vi "NIMS_NS_fir_linf.vi"(5 "Function name":string, 6 "Line number":i32, 7 "Number of outputs requested":i32, 8 "error in (no error)":errorcluster, 11 "[A]":variant[](array[variant])) -> (0 "error out":errorcluster, 3 "[funct(A)]":variant[](array[variant]))   [LabVIEW 2017]
uses:
  <vilib>/imath/engines/lvmath/Functions/Error Handling/error.ctl
  <instcachedir>/0/NIMS_RunTimeType_From StrictType (excl LVString)_1019F277F0A747EDBCA0F6C52CA54500.lvgen/NIMS_RunTimeType_From StrictType (excl LVString)_1019F277F0A747EDBCA0F6C52CA54500_000.vi
  <instcachedir>/0/NIMS_Get Scalar_w Error_1987D997E87247DDAC16EA23A5E9E4FC.lvgen/NIMS_Get Scalar_w Error_1987D997E87247DDAC16EA23A5E9E4FC_000.vi
  <instcachedir>/0/NIMS_Get Any Vector_w Error - Matrix_9FDB8FBE264C42EDBC8FF9BA66C3EF33.lvgen/NIMS_Get Any Vector_w Error - Matrix_9FDB8FBE264C42EDBC8FF9BA66C3EF33_001.vi
  <instcachedir>/0/NIMS_Complex To Real_BE01396FDE034E8E94CEBBA1E368668D.lvgen/NIMS_Complex To Real_BE01396FDE034E8E94CEBBA1E368668D_000.vi
  <instcachedir>/0/NIMS_Get Row Vector_w Error - Matrix_7ECCFA0649AF47C08F6F0C496599EB01.lvgen/NIMS_Get Row Vector_w Error - Matrix_7ECCFA0649AF47C08F6F0C496599EB01_000.vi
  <instcachedir>/0/NIMS_RunTimeType_To Numeric_1CBDAFC4EFAD4045A1DE52278D16738D.lvgen/NIMS_RunTimeType_To Numeric_1CBDAFC4EFAD4045A1DE52278D16738D_000.vi
  <vilib>/addons/Digital Filter Design/NI_DigFilter_MathScript.lvlib
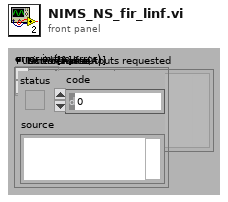
[diagram p1: front panel]
types:
  T1 = typedef "error.ctl" = enum16{"No Error", "Problem", "Input type must not be void", "Incorrect number of parameters", "Function not defined for non-numeric types", "An output variable of the user-defined function is undefined", "Function only defined for character arrays", "Function not defined for boolean, character, or single precision", "Function not defined for complex types", "Not a valid operation", "Inputs must be scalar", "Input matrices are not the same size", "Function only available on RT", "Input matrices must be nonnegative integers of the same type", "Arguments must be non-negative integers less than bitmax", "Number to complement must be less than 2^N", "Bit to get is outside range", "Bit to set is outside range", "Input must be real type ", "At least one parameter must be scalar", "Unable to display plug-in data on RT", "Function not defined for higher dimensional matrices", "Invalid attributes", "Wrong Type of Input Arguments", "Wrong Argument Option", "Invalid file identifier", "Indices must be real positive integers", "The variable is not a matrix data type.", "Number of elements must be the same for indices and values", "You cannot replace elements of a matrix with non-matrix data types.", "Cannot resize a 2D matrix with a linear index", "Unknown variable or symbol", "Indices out of range", "Empty matrix deletion can not be used with two indices", "Number of rows and columns must be the same for indices and values.", "Complex cannot be converted to Boolean", "Char cannot be converted to Boolean", "int64 cannot be converted to Boolean", "uint64 cannot be converted to Boolean", "You cannot convert a Boolean to a character.", "Incompatible input size in 3D surface function", "All rows must have the same number of columns", "Incompatible types", "Invalid matrix dimensions", "Dimension must be 1 or 2", "Base must be an integer between 2 and 36", "Invalid input", "Square matrix required", "Function 'timerstart' must be called before 'timerstop'", "Arguments must be positive real", "Step must not be zero", "Wrong number of input arguments", "Wrong number of output arguments", "Too many index arguments", "Input scalar must be >= 0", "Input scalar must be positive", "Input scalar must not be 0", "Input scalar must be in range [0,1]", "Can't use conditionally defined variable that's undefined", "Input must be a vector", "RT Exec Trace Toolkit not licensed", "Empty vector error", "All elements must be in domain [-1,1]", "All real elements of input vector must be >= 0", "All elements of input vector must be positive", "Values of input vectors are not compatible", "DAQmx not installed", "Input vector must be an increasing vector", "Dereferenced field does not exist within the struct", "A vector or matrix of structures must be indexed before it can be dereferenced", "Lenths of two input vectors are not compatible", "Invalid fieldname", "Empty matrix error", "Cannot use '.' on a type other than Struct", "Unused074", "Data type of the struct's field name is invalid", "Using . to dereference data that is not a struct", "Input struct contains invalid type ", "Size of input matrix is incompatible with input size", "Invalid format specifier", "Could not find field within struct", "Bad permutation array", "Mismatched fieldnames", "ode: User Function could not be opened", "ode: User Function signature does not meet ode requirements", "Unused085", "RunTime: MathScript could not be compiled", "Unknown function", "Only scalars and strings supported", "ode: User Function signature has incorrect number of inputs", "ode:User Function signature has incorrect number of outputs", "Range is too large", "End used without variable", "Function not available (RTE)", "Custom user error", "Arguments must be integers less than bitmax", "Shared library not found", "Header file not found", "Shared library already loaded", "Shared library not loaded", "Shared library function not found", "Shared library string return problem", "Problem calling shared library function", "Problem loading shared library from OS", "Problem parsing shared library header file", "Shared library incompatible types", "Shared library unsupported return type", "Shared library function not exported", "Shared library unsupported input type", "Problem unloading shared library from OS", "Function only available from UI", "Function specified in argument is missing", "An internal error has occurred", "Invalid object", "Invalid property", "Read-only property", "A break command has occurred", "A continue command has occurred", "A return command has occurred", "ode: times parameter invalid", "Function specified in argument has incorrect signature", "Function not found in file", "Reserved keyword cannot be defined as variable", "Reserved keyword cannot be defined as a function or script", "Arguments must be string literals", "Function not supported on this platform", "All columns must have the same number of rows", "Function ignored in RTE warning", "Cannot use : as a parameter that is not a variable", "Output can't be coerced to requested type", "Function not supported on current target", "Variable dependent on an unwired function input", "Unused132", "Unused133", "Unused134", "Unused135", "Unused136", "Unused137", "Unused138", "Unused139", "Global/Persistent must only take constants as arguments.", "Varargin must be last input in the function definition.", "Varargout must be last output in the function definition.", "Invalid output type. Cannot output a cell array of any type other than string.", "Invalid output type. Type is a dynamic struct.", "Invalid output type. Type is a struct that has a field whose type is not known until run-time", "Invalid output type. Type is a struct that has a field which is a plot object.", "MathScript parser DLL missing", "MathScript requires LabVIEW Full", "MathScript license is invalid or missing", "Varargout not supported except in assignments."}
  T2 = typedef "NIMS_CH_character datatype.ctl" = cluster{"Numeric":u8}
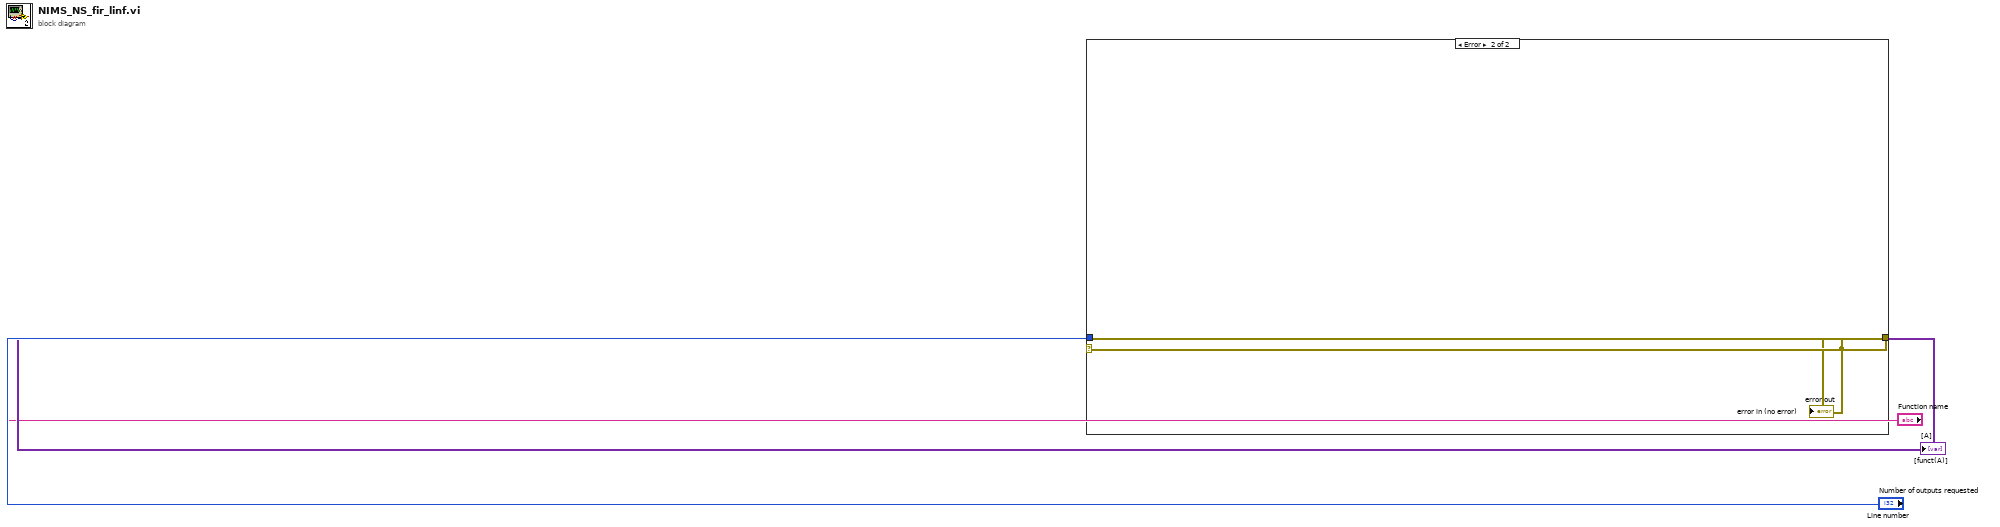
[diagram p0: block diagram]
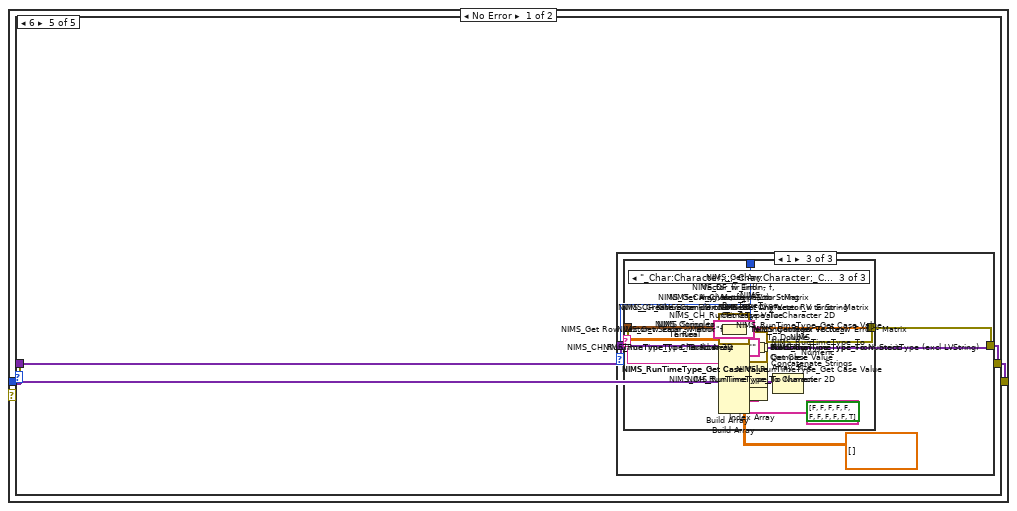
[diagram p2: hidden frame]
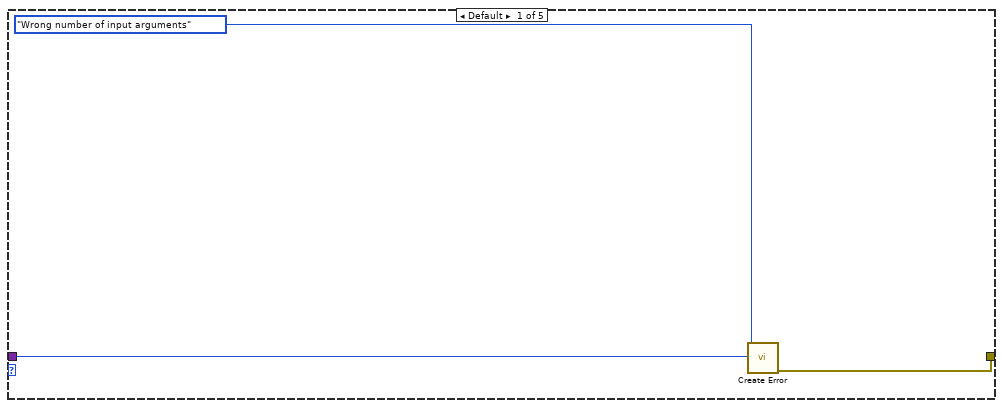
[diagram p3: hidden frame]
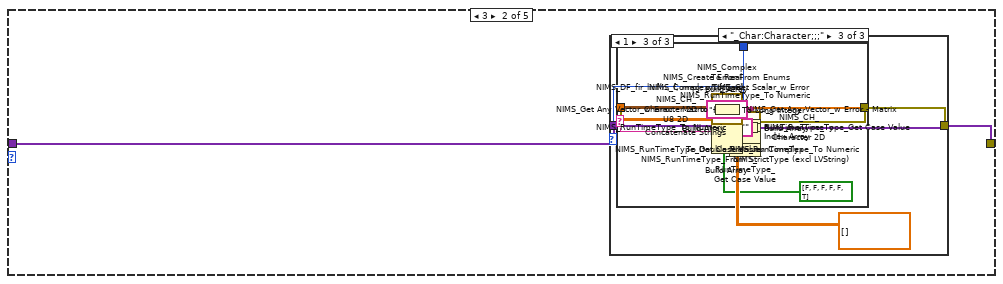
[diagram p4: hidden frame]
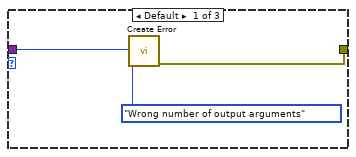
[diagram p5: hidden frame]
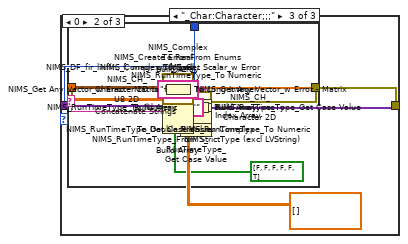
[diagram p6: hidden frame]
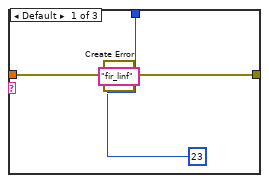
[diagram p7: hidden frame]
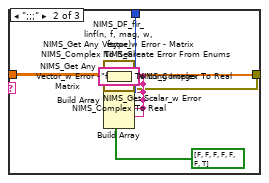
[diagram p8: hidden frame]
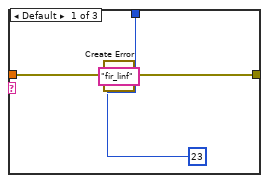
[diagram p9: hidden frame]
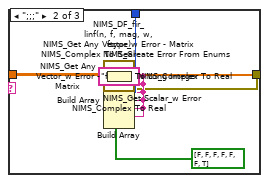
[diagram p10: hidden frame]
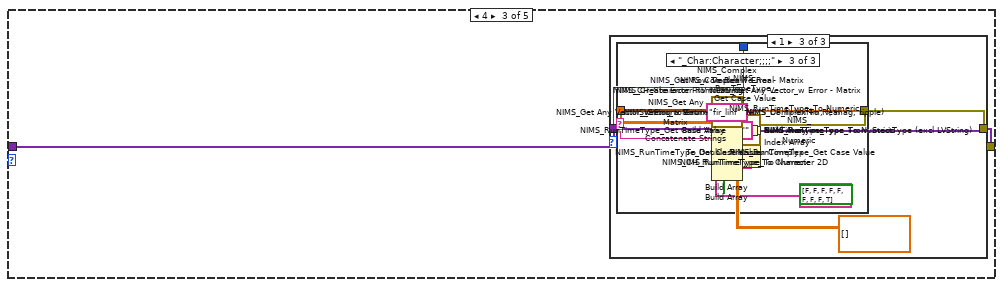
[diagram p11: hidden frame]
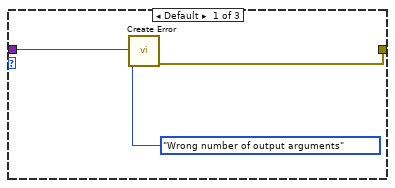
[diagram p12: hidden frame]
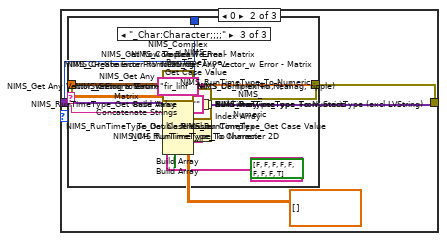
[diagram p13: hidden frame]
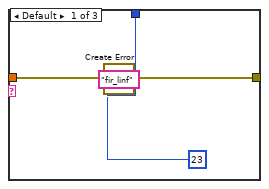
[diagram p14: hidden frame]
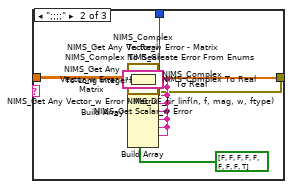
[diagram p15: hidden frame]
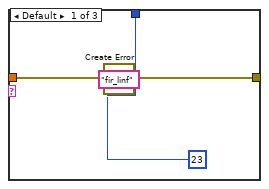
[diagram p16: hidden frame]
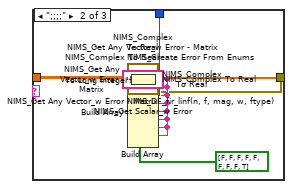
[diagram p17: hidden frame]
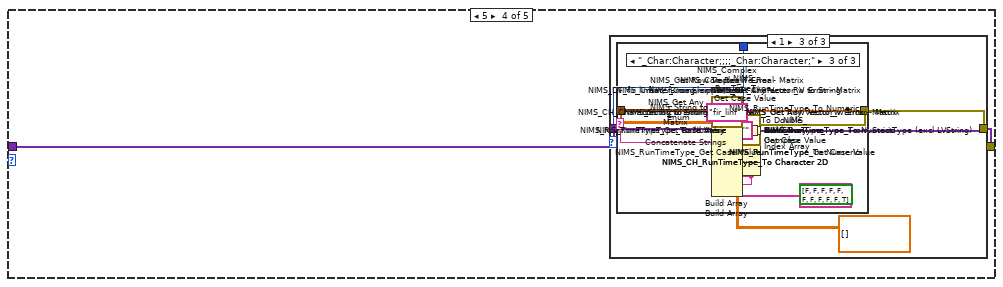
[diagram p18: hidden frame]
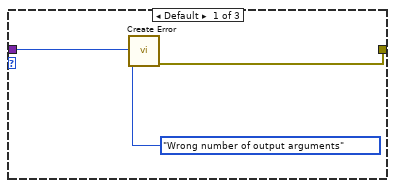
[diagram p19: hidden frame]
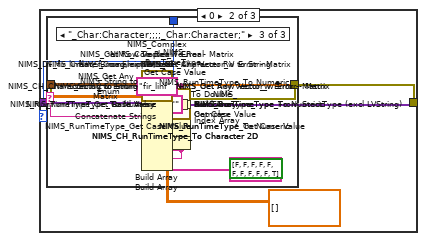
[diagram p20: hidden frame]
diagram:
  n1 = case shown="Error" "error in (no error)" {
    selector: "error in (no error)" -> [_ w885]
    tunnel: [w15 _] -> w4
    tunnel: [w14 w885] -> w3
    tunnel: "error in (no error)" -> [w13 _]
    tunnel: "Number of outputs requested" -> [w12 _]
    tunnel: "[A]" -> [w11 _]
    tunnel: "Function name" -> [w10 _]
    tunnel: "Line number" -> [w9 _]
    frame No Error {
      n2 = Array Size(array=w11) -> (size(s)=w8:i32)
      n3 = case shown="6" w8 {
        tunnel: [_ w27 w199 w403 w635] -> w15
        tunnel: w10 -> [w19 w24 w196 w400 w632]
        tunnel: w9 -> [w20 w25 w197 w401 w633]
        tunnel: w13 -> [w17 w23 w195 w399 w631]
        tunnel: [w16 w22 w194 w398 w630] -> w14
        tunnel: w12 -> [_ w21 w193 w397 w629]
        tunnel: w11 -> [_ w26 w198 w402 w634]
        frame Default {
          n4 = call <vilib>:"Create Error.vi"("Function name"=w19, "error in (no error)"=w17, "Error Enum"=error."Wrong number of input arguments", "Line number"=w20) -> ("error out"=w16:errorcluster)  [unwired: 6 in, 1 out]
        }
        frame 3 {
          n5 = case shown="1" w21 {
            tunnel: [_ w33 w113] -> w27
            tunnel: w24 -> [w31 _ _]
            tunnel: w25 -> [w32 w55 w135]
            tunnel: w23 -> [w29 w53 w133]
            tunnel: [w28 w39 w119] -> w22
            tunnel: w26 -> [_ w56 w136]
            frame Default {
              n6 = call <vilib>:"Create Error.vi"("Function name"=w31, "error in (no error)"=w29, "Error Enum"=error."Wrong number of output arguments", "Line number"=w32) -> ("error out"=w28:errorcluster)  [unwired: 6 in, 1 out]
            }
            frame 0 {
              n7 = Index Array(array=w56) -> (element #1=w52:variant, element #2=w47:variant, element #3=w43:variant)  [unwired: 3 in]
              n8 = call <vilib>:"NIMS_RunTimeType_Get Case Value.vi"("Data In"=w43) -> ("Case Value"=w40:string)  [unwired: 9 in, 1 out]
              n9 = call-generic <vilib>:"NIMS_RunTimeType_To Numeric.vi"("DataType"=cdb[][] [], "Variant"=w43) -> ("data"=w41:cdb[][])  [unwired: 1 in]
              n10 = call <vilib>:"NIMS_RunTimeType_Get Case Value.vi"("Data In"=w47) -> ("Case Value"=w44:string)  [unwired: 9 in, 1 out]
              n11 = call-generic <vilib>:"NIMS_RunTimeType_To Numeric.vi"("DataType"=cdb[][] [], "Variant"=w47) -> ("data"=w45:cdb[][])  [unwired: 1 in]
              n12 = call <vilib>:"NIMS_RunTimeType_Get Case Value.vi"("Data In"=w52) -> ("Case Value"=w48:string)  [unwired: 9 in, 1 out]
              n13 = call <vilib>:"NIMS_CH_RunTimeType_To Character 2D.vi"("Variant"=w52) -> ("data"=w49:T2[][])  [unwired: 1 in]
              n14 = call-generic <vilib>:"NIMS_RunTimeType_To Numeric.vi"("DataType"=cdb[][] [], "Variant"=w52) -> ("data"=w50:cdb[][])  [unwired: 1 in]
              n15 = Concatenate Strings(w48, w44, w40) -> (w54:string)
              n16 = case shown="\"_Char:Character;;;\"" w54 {
                tunnel: w53 -> [w58 w67 w93]
                tunnel: [_ w62 w88] -> w38
                tunnel: [w57 w63 w89] -> w39
                tunnel: w50 -> [_ w86 _]
                tunnel: w49 -> [_ _ w111]
                tunnel: w45 -> [_ w82 w107]
                tunnel: w41 -> [_ w79 w104]
                tunnel: w55 -> [w61 w70 w96]
                frame Default {
                  n17 = call <vilib>:"Create Error.vi"("Function name"="fir_linf", "error in (no error)"=w58, "Error Enum"=23, "Line number"=w61) -> ("error out"=w57:errorcluster)  [unwired: 6 in, 1 out]
                }
                frame ";;;" {
                  w65 = "fir_linf"
                  n18 = call-generic <vilib>:"NIMS_Complex To Real.vi"("A"=w79) -> ("Error Enum"=w73:T1, "Real(A)"=w78:dbl[][])  [unwired: 8 in, 1 out]
                  n19 = call-generic <vilib>:"NIMS_Get Any Vector_w Error - Matrix.vi"("A"=w78) -> ("Error Enum"=w72:T1, "Vector"=w80:dbl[])  [unwired: 8 in, 1 out]
                  n20 = call-generic <vilib>:"NIMS_Complex To Real.vi"("A"=w82) -> ("Error Enum"=w75:T1, "Real(A)"=w81:dbl[][])  [unwired: 8 in, 1 out]
                  n21 = call-generic <vilib>:"NIMS_Get Any Vector_w Error - Matrix.vi"("A"=w81) -> ("Error Enum"=w74:T1, "Vector"=w83:dbl[])  [unwired: 8 in, 1 out]
                  n22 = call-generic <vilib>:"NIMS_Complex To Real.vi"("A"=w86) -> ("Error Enum"=w77:T1, "Real(A)"=w85:dbl[][])  [unwired: 8 in, 1 out]
                  n23 = To Long Integer(number=w85) -> (32bit integer=w84:i32[][])
                  n24 = call-generic <vilib>:"NIMS_Get Scalar_w Error.vi"("A"=w84) -> ("Error Enum"=w76:T1, "Scalar"=w87:i32)  [unwired: 8 in, 1 out]
                  n25 = call <vilib>:"NIMS_DF_fir_linf(n, f, mag, w, ftype).vi"("mag"=w80, "f"=w83, "n"=w87) -> ("error"=w71:i32, "b"=w62:dbl[])  [unwired: 7 in]
                  n26 = Build Array(w65, w65, w65, w65, w65, w65, "fir_linf") -> (w68:string[])
                  n27 = Build Array(w77, w76, w75, w74, w73, w72, w71) -> (w69:i32[])
                  n28 = call <vilib>:"NIMS_Create Error From Enums.vi"("Error Code"=bool[] [FALSE, FALSE, FALSE, FALSE, FALSE, FALSE, TRUE], "error in (no error)"=w67, "Line no"=w70, "Error Enums"=w69, "Function names"=w68) -> ("error out"=w63:errorcluster)  [unwired: 6 in]
                }
                frame "_Char:Character;;;" {
                  w91 = "fir_linf"
                  n29 = call-generic <vilib>:"NIMS_Complex To Real.vi"("A"=w104) -> ("Error Enum"=w99:T1, "Real(A)"=w103:dbl[][])  [unwired: 8 in, 1 out]
                  n30 = call-generic <vilib>:"NIMS_Get Any Vector_w Error - Matrix.vi"("A"=w103) -> ("Error Enum"=w98:T1, "Vector"=w105:dbl[])  [unwired: 8 in, 1 out]
                  n31 = call-generic <vilib>:"NIMS_Complex To Real.vi"("A"=w107) -> ("Error Enum"=w101:T1, "Real(A)"=w106:dbl[][])  [unwired: 8 in, 1 out]
                  n32 = call-generic <vilib>:"NIMS_Get Any Vector_w Error - Matrix.vi"("A"=w106) -> ("Error Enum"=w100:T1, "Vector"=w108:dbl[])  [unwired: 8 in, 1 out]
                  n33 = call <vilib>:"NIMS_CH_Character 2D to U8 2D.vi"("Character 2D array"=w111) -> ("U8 2D array"=w110:u8[][])  [unwired: 10 in]
                  n34 = To Long Integer(number=w110) -> (32bit integer=w109:i32[][])
                  n35 = call-generic <vilib>:"NIMS_Get Scalar_w Error.vi"("A"=w109) -> ("Error Enum"=w102:T1, "Scalar"=w112:i32)  [unwired: 8 in, 1 out]
                  n36 = call <vilib>:"NIMS_DF_fir_linf(n, f, mag, w, ftype).vi"("mag"=w105, "f"=w108, "n"=w112) -> ("error"=w97:i32, "b"=w88:dbl[])  [unwired: 7 in]
                  n37 = Build Array(w91, w91, w91, w91, w91, "fir_linf") -> (w94:string[])
                  n38 = Build Array(w102, w101, w100, w99, w98, w97) -> (w95:i32[])
                  n39 = call <vilib>:"NIMS_Create Error From Enums.vi"("Error Code"=bool[] [FALSE, FALSE, FALSE, FALSE, FALSE, TRUE], "error in (no error)"=w93, "Line no"=w96, "Error Enums"=w95, "Function names"=w94) -> ("error out"=w89:errorcluster)  [unwired: 6 in]
                }
              }
              n40 = Build Array(w38) -> (w37:dbl[][])
              n41 = To Double Precision Complex(1:w37) -> (0:w36:cdb[][])
              n42 = call-generic <vilib>:"NIMS_RunTimeType_From StrictType (excl LVString).vi"("Plug-In Name"="", "Data In"=w36) -> ("Data Out"=w34:variant)  [unwired: 2 in]
              n43 = Build Array(w34) -> (w33:variant[])
            }
            frame 1 {
              n44 = Index Array(array=w136) -> (element #1=w132:variant, element #2=w127:variant, element #3=w123:variant)  [unwired: 3 in]
              n45 = call <vilib>:"NIMS_RunTimeType_Get Case Value.vi"("Data In"=w123) -> ("Case Value"=w120:string)  [unwired: 9 in, 1 out]
              n46 = call-generic <vilib>:"NIMS_RunTimeType_To Numeric.vi"("DataType"=cdb[][] [], "Variant"=w123) -> ("data"=w121:cdb[][])  [unwired: 1 in]
              n47 = call <vilib>:"NIMS_RunTimeType_Get Case Value.vi"("Data In"=w127) -> ("Case Value"=w124:string)  [unwired: 9 in, 1 out]
              n48 = call-generic <vilib>:"NIMS_RunTimeType_To Numeric.vi"("DataType"=cdb[][] [], "Variant"=w127) -> ("data"=w125:cdb[][])  [unwired: 1 in]
              n49 = call <vilib>:"NIMS_RunTimeType_Get Case Value.vi"("Data In"=w132) -> ("Case Value"=w128:string)  [unwired: 9 in, 1 out]
              n50 = call <vilib>:"NIMS_CH_RunTimeType_To Character 2D.vi"("Variant"=w132) -> ("data"=w129:T2[][])  [unwired: 1 in]
              n51 = call-generic <vilib>:"NIMS_RunTimeType_To Numeric.vi"("DataType"=cdb[][] [], "Variant"=w132) -> ("data"=w130:cdb[][])  [unwired: 1 in]
              n52 = Concatenate Strings(w128, w124, w120) -> (w134:string)
              n53 = case shown="\"_Char:Character;;;\"" w134 {
                tunnel: w133 -> [w138 w147 w173]
                tunnel: [_ w142 w168] -> w118
                tunnel: [w137 w143 w169] -> w119
                tunnel: w130 -> [_ w166 _]
                tunnel: w129 -> [_ _ w191]
                tunnel: w125 -> [_ w162 w187]
                tunnel: w121 -> [_ w159 w184]
                tunnel: w135 -> [w141 w150 w176]
                frame Default {
                  n54 = call <vilib>:"Create Error.vi"("Function name"="fir_linf", "error in (no error)"=w138, "Error Enum"=23, "Line number"=w141) -> ("error out"=w137:errorcluster)  [unwired: 6 in, 1 out]
                }
                frame ";;;" {
                  w145 = "fir_linf"
                  n55 = call-generic <vilib>:"NIMS_Complex To Real.vi"("A"=w159) -> ("Error Enum"=w153:T1, "Real(A)"=w158:dbl[][])  [unwired: 8 in, 1 out]
                  n56 = call-generic <vilib>:"NIMS_Get Any Vector_w Error - Matrix.vi"("A"=w158) -> ("Error Enum"=w152:T1, "Vector"=w160:dbl[])  [unwired: 8 in, 1 out]
                  n57 = call-generic <vilib>:"NIMS_Complex To Real.vi"("A"=w162) -> ("Error Enum"=w155:T1, "Real(A)"=w161:dbl[][])  [unwired: 8 in, 1 out]
                  n58 = call-generic <vilib>:"NIMS_Get Any Vector_w Error - Matrix.vi"("A"=w161) -> ("Error Enum"=w154:T1, "Vector"=w163:dbl[])  [unwired: 8 in, 1 out]
                  n59 = call-generic <vilib>:"NIMS_Complex To Real.vi"("A"=w166) -> ("Error Enum"=w157:T1, "Real(A)"=w165:dbl[][])  [unwired: 8 in, 1 out]
                  n60 = To Long Integer(number=w165) -> (32bit integer=w164:i32[][])
                  n61 = call-generic <vilib>:"NIMS_Get Scalar_w Error.vi"("A"=w164) -> ("Error Enum"=w156:T1, "Scalar"=w167:i32)  [unwired: 8 in, 1 out]
                  n62 = call <vilib>:"NIMS_DF_fir_linf(n, f, mag, w, ftype).vi"("mag"=w160, "f"=w163, "n"=w167) -> ("error"=w151:i32, "b"=w142:dbl[])  [unwired: 7 in]
                  n63 = Build Array(w145, w145, w145, w145, w145, w145, "fir_linf") -> (w148:string[])
                  n64 = Build Array(w157, w156, w155, w154, w153, w152, w151) -> (w149:i32[])
                  n65 = call <vilib>:"NIMS_Create Error From Enums.vi"("Error Code"=bool[] [FALSE, FALSE, FALSE, FALSE, FALSE, FALSE, TRUE], "error in (no error)"=w147, "Line no"=w150, "Error Enums"=w149, "Function names"=w148) -> ("error out"=w143:errorcluster)  [unwired: 6 in]
                }
                frame "_Char:Character;;;" {
                  w171 = "fir_linf"
                  n66 = call-generic <vilib>:"NIMS_Complex To Real.vi"("A"=w184) -> ("Error Enum"=w179:T1, "Real(A)"=w183:dbl[][])  [unwired: 8 in, 1 out]
                  n67 = call-generic <vilib>:"NIMS_Get Any Vector_w Error - Matrix.vi"("A"=w183) -> ("Error Enum"=w178:T1, "Vector"=w185:dbl[])  [unwired: 8 in, 1 out]
                  n68 = call-generic <vilib>:"NIMS_Complex To Real.vi"("A"=w187) -> ("Error Enum"=w181:T1, "Real(A)"=w186:dbl[][])  [unwired: 8 in, 1 out]
                  n69 = call-generic <vilib>:"NIMS_Get Any Vector_w Error - Matrix.vi"("A"=w186) -> ("Error Enum"=w180:T1, "Vector"=w188:dbl[])  [unwired: 8 in, 1 out]
                  n70 = call <vilib>:"NIMS_CH_Character 2D to U8 2D.vi"("Character 2D array"=w191) -> ("U8 2D array"=w190:u8[][])  [unwired: 10 in]
                  n71 = To Long Integer(number=w190) -> (32bit integer=w189:i32[][])
                  n72 = call-generic <vilib>:"NIMS_Get Scalar_w Error.vi"("A"=w189) -> ("Error Enum"=w182:T1, "Scalar"=w192:i32)  [unwired: 8 in, 1 out]
                  n73 = call <vilib>:"NIMS_DF_fir_linf(n, f, mag, w, ftype).vi"("mag"=w185, "f"=w188, "n"=w192) -> ("error"=w177:i32, "b"=w168:dbl[])  [unwired: 7 in]
                  n74 = Build Array(w171, w171, w171, w171, w171, "fir_linf") -> (w174:string[])
                  n75 = Build Array(w182, w181, w180, w179, w178, w177) -> (w175:i32[])
                  n76 = call <vilib>:"NIMS_Create Error From Enums.vi"("Error Code"=bool[] [FALSE, FALSE, FALSE, FALSE, FALSE, TRUE], "error in (no error)"=w173, "Line no"=w176, "Error Enums"=w175, "Function names"=w174) -> ("error out"=w169:errorcluster)  [unwired: 6 in]
                }
              }
              n77 = Build Array(w118) -> (w117:dbl[][])
              n78 = To Double Precision Complex(1:w117) -> (0:w116:cdb[][])
              n79 = call-generic <vilib>:"NIMS_RunTimeType_From StrictType (excl LVString).vi"("Plug-In Name"="", "Data In"=w116) -> ("Data Out"=w114:variant)  [unwired: 2 in]
              n80 = Build Array(w114) -> (w113:variant[])
            }
          }
        }
        frame 4 {
          n81 = case shown="1" w193 {
            tunnel: [_ w205 w301] -> w199
            tunnel: w196 -> [w203 _ _]
            tunnel: w197 -> [w204 w231 w327]
            tunnel: w195 -> [w201 w229 w325]
            tunnel: [w200 w211 w307] -> w194
            tunnel: w198 -> [_ w232 w328]
            frame Default {
              n82 = call <vilib>:"Create Error.vi"("Function name"=w203, "error in (no error)"=w201, "Error Enum"=error."Wrong number of output arguments", "Line number"=w204) -> ("error out"=w200:errorcluster)  [unwired: 6 in, 1 out]
            }
            frame 0 {
              n83 = Index Array(array=w232) -> (element #1=w228:variant, element #2=w223:variant, element #3=w219:variant, element #4=w215:variant)  [unwired: 4 in]
              n84 = call <vilib>:"NIMS_RunTimeType_Get Case Value.vi"("Data In"=w215) -> ("Case Value"=w212:string)  [unwired: 9 in, 1 out]
              n85 = call-generic <vilib>:"NIMS_RunTimeType_To Numeric.vi"("DataType"=cdb[][] [], "Variant"=w215) -> ("data"=w213:cdb[][])  [unwired: 1 in]
              n86 = call <vilib>:"NIMS_RunTimeType_Get Case Value.vi"("Data In"=w219) -> ("Case Value"=w216:string)  [unwired: 9 in, 1 out]
              n87 = call-generic <vilib>:"NIMS_RunTimeType_To Numeric.vi"("DataType"=cdb[][] [], "Variant"=w219) -> ("data"=w217:cdb[][])  [unwired: 1 in]
              n88 = call <vilib>:"NIMS_RunTimeType_Get Case Value.vi"("Data In"=w223) -> ("Case Value"=w220:string)  [unwired: 9 in, 1 out]
              n89 = call-generic <vilib>:"NIMS_RunTimeType_To Numeric.vi"("DataType"=cdb[][] [], "Variant"=w223) -> ("data"=w221:cdb[][])  [unwired: 1 in]
              n90 = call <vilib>:"NIMS_RunTimeType_Get Case Value.vi"("Data In"=w228) -> ("Case Value"=w224:string)  [unwired: 9 in, 1 out]
              n91 = call <vilib>:"NIMS_CH_RunTimeType_To Character 2D.vi"("Variant"=w228) -> ("data"=w225:T2[][])  [unwired: 1 in]
              n92 = call-generic <vilib>:"NIMS_RunTimeType_To Numeric.vi"("DataType"=cdb[][] [], "Variant"=w228) -> ("data"=w226:cdb[][])  [unwired: 1 in]
              n93 = Concatenate Strings(w224, w220, w216, w212) -> (w230:string)
              n94 = case shown="\"_Char:Character;;;;\"" w230 {
                tunnel: w229 -> [w234 w243 w274]
                tunnel: [_ w238 w269] -> w210
                tunnel: [w233 w239 w270] -> w211
                tunnel: w226 -> [_ w267 _]
                tunnel: w225 -> [_ _ w298]
                tunnel: w221 -> [_ w263 w294]
                tunnel: w217 -> [_ w260 w291]
                tunnel: w213 -> [_ w257 w288]
                tunnel: w231 -> [w237 w246 w277]
                frame Default {
                  n95 = call <vilib>:"Create Error.vi"("Function name"="fir_linf", "error in (no error)"=w234, "Error Enum"=23, "Line number"=w237) -> ("error out"=w233:errorcluster)  [unwired: 6 in, 1 out]
                }
                frame ";;;;" {
                  w241 = "fir_linf"
                  n96 = call-generic <vilib>:"NIMS_Complex To Real.vi"("A"=w257) -> ("Error Enum"=w249:T1, "Real(A)"=w256:dbl[][])  [unwired: 8 in, 1 out]
                  n97 = call-generic <vilib>:"NIMS_Get Any Vector_w Error - Matrix.vi"("A"=w256) -> ("Error Enum"=w248:T1, "Vector"=w258:dbl[])  [unwired: 8 in, 1 out]
                  n98 = call-generic <vilib>:"NIMS_Complex To Real.vi"("A"=w260) -> ("Error Enum"=w251:T1, "Real(A)"=w259:dbl[][])  [unwired: 8 in, 1 out]
                  n99 = call-generic <vilib>:"NIMS_Get Any Vector_w Error - Matrix.vi"("A"=w259) -> ("Error Enum"=w250:T1, "Vector"=w261:dbl[])  [unwired: 8 in, 1 out]
                  n100 = call-generic <vilib>:"NIMS_Complex To Real.vi"("A"=w263) -> ("Error Enum"=w253:T1, "Real(A)"=w262:dbl[][])  [unwired: 8 in, 1 out]
                  n101 = call-generic <vilib>:"NIMS_Get Any Vector_w Error - Matrix.vi"("A"=w262) -> ("Error Enum"=w252:T1, "Vector"=w264:dbl[])  [unwired: 8 in, 1 out]
                  n102 = call-generic <vilib>:"NIMS_Complex To Real.vi"("A"=w267) -> ("Error Enum"=w255:T1, "Real(A)"=w266:dbl[][])  [unwired: 8 in, 1 out]
                  n103 = To Long Integer(number=w266) -> (32bit integer=w265:i32[][])
                  n104 = call-generic <vilib>:"NIMS_Get Scalar_w Error.vi"("A"=w265) -> ("Error Enum"=w254:T1, "Scalar"=w268:i32)  [unwired: 8 in, 1 out]
                  n105 = call <vilib>:"NIMS_DF_fir_linf(n, f, mag, w, ftype).vi"("w"=w258, "mag"=w261, "f"=w264, "n"=w268) -> ("error"=w247:i32, "b"=w238:dbl[])  [unwired: 6 in]
                  n106 = Build Array(w241, w241, w241, w241, w241, w241, w241, w241, "fir_linf") -> (w244:string[])
                  n107 = Build Array(w255, w254, w253, w252, w251, w250, w249, w248, w247) -> (w245:i32[])
                  n108 = call <vilib>:"NIMS_Create Error From Enums.vi"("Error Code"=bool[] [FALSE, FALSE, FALSE, FALSE, FALSE, FALSE, FALSE, FALSE, TRUE], "error in (no error)"=w243, "Line no"=w246, "Error Enums"=w245, "Function names"=w244) -> ("error out"=w239:errorcluster)  [unwired: 6 in]
                }
                frame "_Char:Character;;;;" {
                  w272 = "fir_linf"
                  n109 = call-generic <vilib>:"NIMS_Complex To Real.vi"("A"=w288) -> ("Error Enum"=w280:T1, "Real(A)"=w287:dbl[][])  [unwired: 8 in, 1 out]
                  n110 = call-generic <vilib>:"NIMS_Get Any Vector_w Error - Matrix.vi"("A"=w287) -> ("Error Enum"=w279:T1, "Vector"=w289:dbl[])  [unwired: 8 in, 1 out]
                  n111 = call-generic <vilib>:"NIMS_Complex To Real.vi"("A"=w291) -> ("Error Enum"=w282:T1, "Real(A)"=w290:dbl[][])  [unwired: 8 in, 1 out]
                  n112 = call-generic <vilib>:"NIMS_Get Any Vector_w Error - Matrix.vi"("A"=w290) -> ("Error Enum"=w281:T1, "Vector"=w292:dbl[])  [unwired: 8 in, 1 out]
                  n113 = call-generic <vilib>:"NIMS_Complex To Real.vi"("A"=w294) -> ("Error Enum"=w284:T1, "Real(A)"=w293:dbl[][])  [unwired: 8 in, 1 out]
                  n114 = call-generic <vilib>:"NIMS_Get Any Vector_w Error - Matrix.vi"("A"=w293) -> ("Error Enum"=w283:T1, "Vector"=w295:dbl[])  [unwired: 8 in, 1 out]
                  n115 = call-generic <vilib>:"NIMS_Get Row Vector_w Error - Matrix.vi"("A"=w298) -> ("Error Enum"=w286:T1, "Row Vector"=w297:T2[])  [unwired: 8 in, 1 out]
                  n116 = call <vilib>:"NIMS_CH_Character RV to String.vi"("Character array"=w297) -> ("String"=w299:string)  [unwired: 10 in]
                  n117 = call <vilib>:"NIMS_String to Enum.vi"("Input String"=w299, "Enum choices"=string[] ["mineven", "minodd"] ("Enum Options")) -> ("Error Enum"=w285:T1, "Enum Index"=w300:i32)  [unwired: 8 in]
                  n118 = call <vilib>:"NIMS_DF_fir_linf(m, f, mag, ripple).vi"("ripple"=w289, "mag"=w292, "f"=w295, "flag"=w300) -> ("error"=w278:i32, "b"=w269:dbl[])  [unwired: 6 in]
                  n119 = Build Array(w272, w272, w272, w272, w272, w272, w272, w272, "fir_linf") -> (w275:string[])
                  n120 = Build Array(w286, w285, w284, w283, w282, w281, w280, w279, w278) -> (w276:i32[])
                  n121 = call <vilib>:"NIMS_Create Error From Enums.vi"("Error Code"=bool[] [FALSE, FALSE, FALSE, FALSE, FALSE, FALSE, FALSE, FALSE, TRUE], "error in (no error)"=w274, "Line no"=w277, "Error Enums"=w276, "Function names"=w275) -> ("error out"=w270:errorcluster)  [unwired: 6 in]
                }
              }
              n122 = Build Array(w210) -> (w209:dbl[][])
              n123 = To Double Precision Complex(1:w209) -> (0:w208:cdb[][])
              n124 = call-generic <vilib>:"NIMS_RunTimeType_From StrictType (excl LVString).vi"("Plug-In Name"="", "Data In"=w208) -> ("Data Out"=w206:variant)  [unwired: 2 in]
              n125 = Build Array(w206) -> (w205:variant[])
            }
            frame 1 {
              n126 = Index Array(array=w328) -> (element #1=w324:variant, element #2=w319:variant, element #3=w315:variant, element #4=w311:variant)  [unwired: 4 in]
              n127 = call <vilib>:"NIMS_RunTimeType_Get Case Value.vi"("Data In"=w311) -> ("Case Value"=w308:string)  [unwired: 9 in, 1 out]
              n128 = call-generic <vilib>:"NIMS_RunTimeType_To Numeric.vi"("DataType"=cdb[][] [], "Variant"=w311) -> ("data"=w309:cdb[][])  [unwired: 1 in]
              n129 = call <vilib>:"NIMS_RunTimeType_Get Case Value.vi"("Data In"=w315) -> ("Case Value"=w312:string)  [unwired: 9 in, 1 out]
              n130 = call-generic <vilib>:"NIMS_RunTimeType_To Numeric.vi"("DataType"=cdb[][] [], "Variant"=w315) -> ("data"=w313:cdb[][])  [unwired: 1 in]
              n131 = call <vilib>:"NIMS_RunTimeType_Get Case Value.vi"("Data In"=w319) -> ("Case Value"=w316:string)  [unwired: 9 in, 1 out]
              n132 = call-generic <vilib>:"NIMS_RunTimeType_To Numeric.vi"("DataType"=cdb[][] [], "Variant"=w319) -> ("data"=w317:cdb[][])  [unwired: 1 in]
              n133 = call <vilib>:"NIMS_RunTimeType_Get Case Value.vi"("Data In"=w324) -> ("Case Value"=w320:string)  [unwired: 9 in, 1 out]
              n134 = call <vilib>:"NIMS_CH_RunTimeType_To Character 2D.vi"("Variant"=w324) -> ("data"=w321:T2[][])  [unwired: 1 in]
              n135 = call-generic <vilib>:"NIMS_RunTimeType_To Numeric.vi"("DataType"=cdb[][] [], "Variant"=w324) -> ("data"=w322:cdb[][])  [unwired: 1 in]
              n136 = Concatenate Strings(w320, w316, w312, w308) -> (w326:string)
              n137 = case shown="\"_Char:Character;;;;\"" w326 {
                tunnel: w325 -> [w330 w339 w370]
                tunnel: [_ w334 w365] -> w306
                tunnel: [w329 w335 w366] -> w307
                tunnel: w322 -> [_ w363 _]
                tunnel: w321 -> [_ _ w394]
                tunnel: w317 -> [_ w359 w390]
                tunnel: w313 -> [_ w356 w387]
                tunnel: w309 -> [_ w353 w384]
                tunnel: w327 -> [w333 w342 w373]
                frame Default {
                  n138 = call <vilib>:"Create Error.vi"("Function name"="fir_linf", "error in (no error)"=w330, "Error Enum"=23, "Line number"=w333) -> ("error out"=w329:errorcluster)  [unwired: 6 in, 1 out]
                }
                frame ";;;;" {
                  w337 = "fir_linf"
                  n139 = call-generic <vilib>:"NIMS_Complex To Real.vi"("A"=w353) -> ("Error Enum"=w345:T1, "Real(A)"=w352:dbl[][])  [unwired: 8 in, 1 out]
                  n140 = call-generic <vilib>:"NIMS_Get Any Vector_w Error - Matrix.vi"("A"=w352) -> ("Error Enum"=w344:T1, "Vector"=w354:dbl[])  [unwired: 8 in, 1 out]
                  n141 = call-generic <vilib>:"NIMS_Complex To Real.vi"("A"=w356) -> ("Error Enum"=w347:T1, "Real(A)"=w355:dbl[][])  [unwired: 8 in, 1 out]
                  n142 = call-generic <vilib>:"NIMS_Get Any Vector_w Error - Matrix.vi"("A"=w355) -> ("Error Enum"=w346:T1, "Vector"=w357:dbl[])  [unwired: 8 in, 1 out]
                  n143 = call-generic <vilib>:"NIMS_Complex To Real.vi"("A"=w359) -> ("Error Enum"=w349:T1, "Real(A)"=w358:dbl[][])  [unwired: 8 in, 1 out]
                  n144 = call-generic <vilib>:"NIMS_Get Any Vector_w Error - Matrix.vi"("A"=w358) -> ("Error Enum"=w348:T1, "Vector"=w360:dbl[])  [unwired: 8 in, 1 out]
                  n145 = call-generic <vilib>:"NIMS_Complex To Real.vi"("A"=w363) -> ("Error Enum"=w351:T1, "Real(A)"=w362:dbl[][])  [unwired: 8 in, 1 out]
                  n146 = To Long Integer(number=w362) -> (32bit integer=w361:i32[][])
                  n147 = call-generic <vilib>:"NIMS_Get Scalar_w Error.vi"("A"=w361) -> ("Error Enum"=w350:T1, "Scalar"=w364:i32)  [unwired: 8 in, 1 out]
                  n148 = call <vilib>:"NIMS_DF_fir_linf(n, f, mag, w, ftype).vi"("w"=w354, "mag"=w357, "f"=w360, "n"=w364) -> ("error"=w343:i32, "b"=w334:dbl[])  [unwired: 6 in]
                  n149 = Build Array(w337, w337, w337, w337, w337, w337, w337, w337, "fir_linf") -> (w340:string[])
                  n150 = Build Array(w351, w350, w349, w348, w347, w346, w345, w344, w343) -> (w341:i32[])
                  n151 = call <vilib>:"NIMS_Create Error From Enums.vi"("Error Code"=bool[] [FALSE, FALSE, FALSE, FALSE, FALSE, FALSE, FALSE, FALSE, TRUE], "error in (no error)"=w339, "Line no"=w342, "Error Enums"=w341, "Function names"=w340) -> ("error out"=w335:errorcluster)  [unwired: 6 in]
                }
                frame "_Char:Character;;;;" {
                  w368 = "fir_linf"
                  n152 = call-generic <vilib>:"NIMS_Complex To Real.vi"("A"=w384) -> ("Error Enum"=w376:T1, "Real(A)"=w383:dbl[][])  [unwired: 8 in, 1 out]
                  n153 = call-generic <vilib>:"NIMS_Get Any Vector_w Error - Matrix.vi"("A"=w383) -> ("Error Enum"=w375:T1, "Vector"=w385:dbl[])  [unwired: 8 in, 1 out]
                  n154 = call-generic <vilib>:"NIMS_Complex To Real.vi"("A"=w387) -> ("Error Enum"=w378:T1, "Real(A)"=w386:dbl[][])  [unwired: 8 in, 1 out]
                  n155 = call-generic <vilib>:"NIMS_Get Any Vector_w Error - Matrix.vi"("A"=w386) -> ("Error Enum"=w377:T1, "Vector"=w388:dbl[])  [unwired: 8 in, 1 out]
                  n156 = call-generic <vilib>:"NIMS_Complex To Real.vi"("A"=w390) -> ("Error Enum"=w380:T1, "Real(A)"=w389:dbl[][])  [unwired: 8 in, 1 out]
                  n157 = call-generic <vilib>:"NIMS_Get Any Vector_w Error - Matrix.vi"("A"=w389) -> ("Error Enum"=w379:T1, "Vector"=w391:dbl[])  [unwired: 8 in, 1 out]
                  n158 = call-generic <vilib>:"NIMS_Get Row Vector_w Error - Matrix.vi"("A"=w394) -> ("Error Enum"=w382:T1, "Row Vector"=w393:T2[])  [unwired: 8 in, 1 out]
                  n159 = call <vilib>:"NIMS_CH_Character RV to String.vi"("Character array"=w393) -> ("String"=w395:string)  [unwired: 10 in]
                  n160 = call <vilib>:"NIMS_String to Enum.vi"("Input String"=w395, "Enum choices"=string[] ["mineven", "minodd"] ("Enum Options")) -> ("Error Enum"=w381:T1, "Enum Index"=w396:i32)  [unwired: 8 in]
                  n161 = call <vilib>:"NIMS_DF_fir_linf(m, f, mag, ripple).vi"("ripple"=w385, "mag"=w388, "f"=w391, "flag"=w396) -> ("error"=w374:i32, "b"=w365:dbl[])  [unwired: 6 in]
                  n162 = Build Array(w368, w368, w368, w368, w368, w368, w368, w368, "fir_linf") -> (w371:string[])
                  n163 = Build Array(w382, w381, w380, w379, w378, w377, w376, w375, w374) -> (w372:i32[])
                  n164 = call <vilib>:"NIMS_Create Error From Enums.vi"("Error Code"=bool[] [FALSE, FALSE, FALSE, FALSE, FALSE, FALSE, FALSE, FALSE, TRUE], "error in (no error)"=w370, "Line no"=w373, "Error Enums"=w372, "Function names"=w371) -> ("error out"=w366:errorcluster)  [unwired: 6 in]
                }
              }
              n165 = Build Array(w306) -> (w305:dbl[][])
              n166 = To Double Precision Complex(1:w305) -> (0:w304:cdb[][])
              n167 = call-generic <vilib>:"NIMS_RunTimeType_From StrictType (excl LVString).vi"("Plug-In Name"="", "Data In"=w304) -> ("Data Out"=w302:variant)  [unwired: 2 in]
              n168 = Build Array(w302) -> (w301:variant[])
            }
          }
        }
        frame 5 {
          n169 = case shown="1" w397 {
            tunnel: [_ w409 w519] -> w403
            tunnel: w400 -> [w407 _ _]
            tunnel: w401 -> [w408 w438 w548]
            tunnel: w399 -> [w405 w436 w546]
            tunnel: [w404 w415 w525] -> w398
            tunnel: w402 -> [_ w439 w549]
            frame Default {
              n170 = call <vilib>:"Create Error.vi"("Function name"=w407, "error in (no error)"=w405, "Error Enum"=error."Wrong number of output arguments", "Line number"=w408) -> ("error out"=w404:errorcluster)  [unwired: 6 in, 1 out]
            }
            frame 0 {
              n171 = Index Array(array=w439) -> (element #1=w435:variant, element #2=w430:variant, element #3=w426:variant, element #4=w422:variant, element #5=w418:variant)  [unwired: 5 in]
              n172 = call <vilib>:"NIMS_RunTimeType_Get Case Value.vi"("Data In"=w418) -> ("Case Value"=w416:string)  [unwired: 9 in, 1 out]
              n173 = call <vilib>:"NIMS_CH_RunTimeType_To Character 2D.vi"("Variant"=w418) -> ("data"=w417:T2[][])  [unwired: 1 in]
              n174 = call <vilib>:"NIMS_RunTimeType_Get Case Value.vi"("Data In"=w422) -> ("Case Value"=w419:string)  [unwired: 9 in, 1 out]
              n175 = call-generic <vilib>:"NIMS_RunTimeType_To Numeric.vi"("DataType"=cdb[][] [], "Variant"=w422) -> ("data"=w420:cdb[][])  [unwired: 1 in]
              n176 = call <vilib>:"NIMS_RunTimeType_Get Case Value.vi"("Data In"=w426) -> ("Case Value"=w423:string)  [unwired: 9 in, 1 out]
              n177 = call-generic <vilib>:"NIMS_RunTimeType_To Numeric.vi"("DataType"=cdb[][] [], "Variant"=w426) -> ("data"=w424:cdb[][])  [unwired: 1 in]
              n178 = call <vilib>:"NIMS_RunTimeType_Get Case Value.vi"("Data In"=w430) -> ("Case Value"=w427:string)  [unwired: 9 in, 1 out]
              n179 = call-generic <vilib>:"NIMS_RunTimeType_To Numeric.vi"("DataType"=cdb[][] [], "Variant"=w430) -> ("data"=w428:cdb[][])  [unwired: 1 in]
              n180 = call <vilib>:"NIMS_RunTimeType_Get Case Value.vi"("Data In"=w435) -> ("Case Value"=w431:string)  [unwired: 9 in, 1 out]
              n181 = call <vilib>:"NIMS_CH_RunTimeType_To Character 2D.vi"("Variant"=w435) -> ("data"=w432:T2[][])  [unwired: 1 in]
              n182 = call-generic <vilib>:"NIMS_RunTimeType_To Numeric.vi"("DataType"=cdb[][] [], "Variant"=w435) -> ("data"=w433:cdb[][])  [unwired: 1 in]
              n183 = Concatenate Strings(w431, w427, w423, w419, w416) -> (w437:string)
              n184 = case shown="\"_Char:Character;;;;_Char:Character;\"" w437 {
                tunnel: w436 -> [w441 w450 w485]
                tunnel: [_ w445 w480] -> w414
                tunnel: [w440 w446 w481] -> w415
                tunnel: w433 -> [_ w478 _]
                tunnel: w432 -> [_ _ w516]
                tunnel: w428 -> [_ w474 w512]
                tunnel: w424 -> [_ w471 w509]
                tunnel: w420 -> [_ w468 w506]
                tunnel: w417 -> [_ w465 w502]
                tunnel: w438 -> [w444 w453 w488]
                frame Default {
                  n185 = call <vilib>:"Create Error.vi"("Function name"="fir_linf", "error in (no error)"=w441, "Error Enum"=23, "Line number"=w444) -> ("error out"=w440:errorcluster)  [unwired: 6 in, 1 out]
                }
                frame ";;;;_Char:Character;" {
                  w448 = "fir_linf"
                  n186 = call-generic <vilib>:"NIMS_Get Row Vector_w Error - Matrix.vi"("A"=w465) -> ("Error Enum"=w455:T1, "Row Vector"=w464:T2[])  [unwired: 8 in, 1 out]
                  n187 = call <vilib>:"NIMS_CH_Character RV to String.vi"("Character array"=w464) -> ("String"=w466:string)  [unwired: 10 in]
                  n188 = call-generic <vilib>:"NIMS_Complex To Real.vi"("A"=w468) -> ("Error Enum"=w457:T1, "Real(A)"=w467:dbl[][])  [unwired: 8 in, 1 out]
                  n189 = call-generic <vilib>:"NIMS_Get Any Vector_w Error - Matrix.vi"("A"=w467) -> ("Error Enum"=w456:T1, "Vector"=w469:dbl[])  [unwired: 8 in, 1 out]
                  n190 = call-generic <vilib>:"NIMS_Complex To Real.vi"("A"=w471) -> ("Error Enum"=w459:T1, "Real(A)"=w470:dbl[][])  [unwired: 8 in, 1 out]
                  n191 = call-generic <vilib>:"NIMS_Get Any Vector_w Error - Matrix.vi"("A"=w470) -> ("Error Enum"=w458:T1, "Vector"=w472:dbl[])  [unwired: 8 in, 1 out]
                  n192 = call-generic <vilib>:"NIMS_Complex To Real.vi"("A"=w474) -> ("Error Enum"=w461:T1, "Real(A)"=w473:dbl[][])  [unwired: 8 in, 1 out]
                  n193 = call-generic <vilib>:"NIMS_Get Any Vector_w Error - Matrix.vi"("A"=w473) -> ("Error Enum"=w460:T1, "Vector"=w475:dbl[])  [unwired: 8 in, 1 out]
                  n194 = call-generic <vilib>:"NIMS_Complex To Real.vi"("A"=w478) -> ("Error Enum"=w463:T1, "Real(A)"=w477:dbl[][])  [unwired: 8 in, 1 out]
                  n195 = To Long Integer(number=w477) -> (32bit integer=w476:i32[][])
                  n196 = call-generic <vilib>:"NIMS_Get Scalar_w Error.vi"("A"=w476) -> ("Error Enum"=w462:T1, "Scalar"=w479:i32)  [unwired: 8 in, 1 out]
                  n197 = call <vilib>:"NIMS_DF_fir_linf(n, f, mag, w, ftype).vi"("ftype"=w466, "w"=w469, "mag"=w472, "f"=w475, "n"=w479) -> ("error"=w454:i32, "b"=w445:dbl[])  [unwired: 5 in]
                  n198 = Build Array(w448, w448, w448, w448, w448, w448, w448, w448, w448, "fir_linf") -> (w451:string[])
                  n199 = Build Array(w463, w462, w461, w460, w459, w458, w457, w456, w455, w454) -> (w452:i32[])
                  n200 = call <vilib>:"NIMS_Create Error From Enums.vi"("Error Code"=bool[] [FALSE, FALSE, FALSE, FALSE, FALSE, FALSE, FALSE, FALSE, FALSE, TRUE], "error in (no error)"=w450, "Line no"=w453, "Error Enums"=w452, "Function names"=w451) -> ("error out"=w446:errorcluster)  [unwired: 6 in]
                }
                frame "_Char:Character;;;;_Char:Character;" {
                  w483 = "fir_linf"
                  n201 = call-generic <vilib>:"NIMS_Get Row Vector_w Error - Matrix.vi"("A"=w502) -> ("Error Enum"=w491:T1, "Row Vector"=w501:T2[])  [unwired: 8 in, 1 out]
                  n202 = call <vilib>:"NIMS_CH_Character RV to String.vi"("Character array"=w501) -> ("String"=w503:string)  [unwired: 10 in]
                  n203 = call <vilib>:"NIMS_String to Enum.vi"("Input String"=w503, "Enum choices"=string[] ["Type I", "Type II", "Type III", "Type IV"] ("Enum Options")) -> ("Error Enum"=w490:T1, "Enum Index"=w504:i32)  [unwired: 8 in]
                  n204 = call-generic <vilib>:"NIMS_Complex To Real.vi"("A"=w506) -> ("Error Enum"=w493:T1, "Real(A)"=w505:dbl[][])  [unwired: 8 in, 1 out]
                  n205 = call-generic <vilib>:"NIMS_Get Any Vector_w Error - Matrix.vi"("A"=w505) -> ("Error Enum"=w492:T1, "Vector"=w507:dbl[])  [unwired: 8 in, 1 out]
                  n206 = call-generic <vilib>:"NIMS_Complex To Real.vi"("A"=w509) -> ("Error Enum"=w495:T1, "Real(A)"=w508:dbl[][])  [unwired: 8 in, 1 out]
                  n207 = call-generic <vilib>:"NIMS_Get Any Vector_w Error - Matrix.vi"("A"=w508) -> ("Error Enum"=w494:T1, "Vector"=w510:dbl[])  [unwired: 8 in, 1 out]
                  n208 = call-generic <vilib>:"NIMS_Complex To Real.vi"("A"=w512) -> ("Error Enum"=w497:T1, "Real(A)"=w511:dbl[][])  [unwired: 8 in, 1 out]
                  n209 = call-generic <vilib>:"NIMS_Get Any Vector_w Error - Matrix.vi"("A"=w511) -> ("Error Enum"=w496:T1, "Vector"=w513:dbl[])  [unwired: 8 in, 1 out]
                  n210 = call-generic <vilib>:"NIMS_Get Row Vector_w Error - Matrix.vi"("A"=w516) -> ("Error Enum"=w499:T1, "Row Vector"=w515:T2[])  [unwired: 8 in, 1 out]
                  n211 = call <vilib>:"NIMS_CH_Character RV to String.vi"("Character array"=w515) -> ("String"=w517:string)  [unwired: 10 in]
                  n212 = call <vilib>:"NIMS_String to Enum.vi"("Input String"=w517, "Enum choices"=string[] ["minorder"] ("Enum Options")) -> ("Error Enum"=w498:T1, "Enum Index"=w518:i32)  [unwired: 8 in]
                  n213 = call <vilib>:"NIMS_DF_fir_linf(m, f, mag, ripple, tm).vi"("type"=w504, "ripple"=w507, "mag"=w510, "f"=w513, "flag"=w518) -> ("error"=w489:i32, "b"=w480:dbl[])  [unwired: 5 in]
                  n214 = Build Array(w483, w483, w483, w483, w483, w483, w483, w483, w483, w483, "fir_linf") -> (w486:string[])
                  n215 = Build Array(w499, w498, w497, w496, w495, w494, w493, w492, w491, w490, w489) -> (w487:i32[])
                  n216 = call <vilib>:"NIMS_Create Error From Enums.vi"("Error Code"=bool[] [FALSE, FALSE, FALSE, FALSE, FALSE, FALSE, FALSE, FALSE, FALSE, FALSE, TRUE], "error in (no error)"=w485, "Line no"=w488, "Error Enums"=w487, "Function names"=w486) -> ("error out"=w481:errorcluster)  [unwired: 6 in]
                }
              }
              n217 = Build Array(w414) -> (w413:dbl[][])
              n218 = To Double Precision Complex(1:w413) -> (0:w412:cdb[][])
              n219 = call-generic <vilib>:"NIMS_RunTimeType_From StrictType (excl LVString).vi"("Plug-In Name"="", "Data In"=w412) -> ("Data Out"=w410:variant)  [unwired: 2 in]
              n220 = Build Array(w410) -> (w409:variant[])
            }
            frame 1 {
              n221 = Index Array(array=w549) -> (element #1=w545:variant, element #2=w540:variant, element #3=w536:variant, element #4=w532:variant, element #5=w528:variant)  [unwired: 5 in]
              n222 = call <vilib>:"NIMS_RunTimeType_Get Case Value.vi"("Data In"=w528) -> ("Case Value"=w526:string)  [unwired: 9 in, 1 out]
              n223 = call <vilib>:"NIMS_CH_RunTimeType_To Character 2D.vi"("Variant"=w528) -> ("data"=w527:T2[][])  [unwired: 1 in]
              n224 = call <vilib>:"NIMS_RunTimeType_Get Case Value.vi"("Data In"=w532) -> ("Case Value"=w529:string)  [unwired: 9 in, 1 out]
              n225 = call-generic <vilib>:"NIMS_RunTimeType_To Numeric.vi"("DataType"=cdb[][] [], "Variant"=w532) -> ("data"=w530:cdb[][])  [unwired: 1 in]
              n226 = call <vilib>:"NIMS_RunTimeType_Get Case Value.vi"("Data In"=w536) -> ("Case Value"=w533:string)  [unwired: 9 in, 1 out]
              n227 = call-generic <vilib>:"NIMS_RunTimeType_To Numeric.vi"("DataType"=cdb[][] [], "Variant"=w536) -> ("data"=w534:cdb[][])  [unwired: 1 in]
              n228 = call <vilib>:"NIMS_RunTimeType_Get Case Value.vi"("Data In"=w540) -> ("Case Value"=w537:string)  [unwired: 9 in, 1 out]
              n229 = call-generic <vilib>:"NIMS_RunTimeType_To Numeric.vi"("DataType"=cdb[][] [], "Variant"=w540) -> ("data"=w538:cdb[][])  [unwired: 1 in]
              n230 = call <vilib>:"NIMS_RunTimeType_Get Case Value.vi"("Data In"=w545) -> ("Case Value"=w541:string)  [unwired: 9 in, 1 out]
              n231 = call <vilib>:"NIMS_CH_RunTimeType_To Character 2D.vi"("Variant"=w545) -> ("data"=w542:T2[][])  [unwired: 1 in]
              n232 = call-generic <vilib>:"NIMS_RunTimeType_To Numeric.vi"("DataType"=cdb[][] [], "Variant"=w545) -> ("data"=w543:cdb[][])  [unwired: 1 in]
              n233 = Concatenate Strings(w541, w537, w533, w529, w526) -> (w547:string)
              n234 = case shown="\"_Char:Character;;;;_Char:Character;\"" w547 {
                tunnel: w546 -> [w551 w560 w595]
                tunnel: [_ w555 w590] -> w524
                tunnel: [w550 w556 w591] -> w525
                tunnel: w543 -> [_ w588 _]
                tunnel: w542 -> [_ _ w626]
                tunnel: w538 -> [_ w584 w622]
                tunnel: w534 -> [_ w581 w619]
                tunnel: w530 -> [_ w578 w616]
                tunnel: w527 -> [_ w575 w612]
                tunnel: w548 -> [w554 w563 w598]
                frame Default {
                  n235 = call <vilib>:"Create Error.vi"("Function name"="fir_linf", "error in (no error)"=w551, "Error Enum"=23, "Line number"=w554) -> ("error out"=w550:errorcluster)  [unwired: 6 in, 1 out]
                }
                frame ";;;;_Char:Character;" {
                  w558 = "fir_linf"
                  n236 = call-generic <vilib>:"NIMS_Get Row Vector_w Error - Matrix.vi"("A"=w575) -> ("Error Enum"=w565:T1, "Row Vector"=w574:T2[])  [unwired: 8 in, 1 out]
                  n237 = call <vilib>:"NIMS_CH_Character RV to String.vi"("Character array"=w574) -> ("String"=w576:string)  [unwired: 10 in]
                  n238 = call-generic <vilib>:"NIMS_Complex To Real.vi"("A"=w578) -> ("Error Enum"=w567:T1, "Real(A)"=w577:dbl[][])  [unwired: 8 in, 1 out]
                  n239 = call-generic <vilib>:"NIMS_Get Any Vector_w Error - Matrix.vi"("A"=w577) -> ("Error Enum"=w566:T1, "Vector"=w579:dbl[])  [unwired: 8 in, 1 out]
                  n240 = call-generic <vilib>:"NIMS_Complex To Real.vi"("A"=w581) -> ("Error Enum"=w569:T1, "Real(A)"=w580:dbl[][])  [unwired: 8 in, 1 out]
                  n241 = call-generic <vilib>:"NIMS_Get Any Vector_w Error - Matrix.vi"("A"=w580) -> ("Error Enum"=w568:T1, "Vector"=w582:dbl[])  [unwired: 8 in, 1 out]
                  n242 = call-generic <vilib>:"NIMS_Complex To Real.vi"("A"=w584) -> ("Error Enum"=w571:T1, "Real(A)"=w583:dbl[][])  [unwired: 8 in, 1 out]
                  n243 = call-generic <vilib>:"NIMS_Get Any Vector_w Error - Matrix.vi"("A"=w583) -> ("Error Enum"=w570:T1, "Vector"=w585:dbl[])  [unwired: 8 in, 1 out]
                  n244 = call-generic <vilib>:"NIMS_Complex To Real.vi"("A"=w588) -> ("Error Enum"=w573:T1, "Real(A)"=w587:dbl[][])  [unwired: 8 in, 1 out]
                  n245 = To Long Integer(number=w587) -> (32bit integer=w586:i32[][])
                  n246 = call-generic <vilib>:"NIMS_Get Scalar_w Error.vi"("A"=w586) -> ("Error Enum"=w572:T1, "Scalar"=w589:i32)  [unwired: 8 in, 1 out]
                  n247 = call <vilib>:"NIMS_DF_fir_linf(n, f, mag, w, ftype).vi"("ftype"=w576, "w"=w579, "mag"=w582, "f"=w585, "n"=w589) -> ("error"=w564:i32, "b"=w555:dbl[])  [unwired: 5 in]
                  n248 = Build Array(w558, w558, w558, w558, w558, w558, w558, w558, w558, "fir_linf") -> (w561:string[])
                  n249 = Build Array(w573, w572, w571, w570, w569, w568, w567, w566, w565, w564) -> (w562:i32[])
                  n250 = call <vilib>:"NIMS_Create Error From Enums.vi"("Error Code"=bool[] [FALSE, FALSE, FALSE, FALSE, FALSE, FALSE, FALSE, FALSE, FALSE, TRUE], "error in (no error)"=w560, "Line no"=w563, "Error Enums"=w562, "Function names"=w561) -> ("error out"=w556:errorcluster)  [unwired: 6 in]
                }
                frame "_Char:Character;;;;_Char:Character;" {
                  w593 = "fir_linf"
                  n251 = call-generic <vilib>:"NIMS_Get Row Vector_w Error - Matrix.vi"("A"=w612) -> ("Error Enum"=w601:T1, "Row Vector"=w611:T2[])  [unwired: 8 in, 1 out]
                  n252 = call <vilib>:"NIMS_CH_Character RV to String.vi"("Character array"=w611) -> ("String"=w613:string)  [unwired: 10 in]
                  n253 = call <vilib>:"NIMS_String to Enum.vi"("Input String"=w613, "Enum choices"=string[] ["Type I", "Type II", "Type III", "Type IV"] ("Enum Options")) -> ("Error Enum"=w600:T1, "Enum Index"=w614:i32)  [unwired: 8 in]
                  n254 = call-generic <vilib>:"NIMS_Complex To Real.vi"("A"=w616) -> ("Error Enum"=w603:T1, "Real(A)"=w615:dbl[][])  [unwired: 8 in, 1 out]
                  n255 = call-generic <vilib>:"NIMS_Get Any Vector_w Error - Matrix.vi"("A"=w615) -> ("Error Enum"=w602:T1, "Vector"=w617:dbl[])  [unwired: 8 in, 1 out]
                  n256 = call-generic <vilib>:"NIMS_Complex To Real.vi"("A"=w619) -> ("Error Enum"=w605:T1, "Real(A)"=w618:dbl[][])  [unwired: 8 in, 1 out]
                  n257 = call-generic <vilib>:"NIMS_Get Any Vector_w Error - Matrix.vi"("A"=w618) -> ("Error Enum"=w604:T1, "Vector"=w620:dbl[])  [unwired: 8 in, 1 out]
                  n258 = call-generic <vilib>:"NIMS_Complex To Real.vi"("A"=w622) -> ("Error Enum"=w607:T1, "Real(A)"=w621:dbl[][])  [unwired: 8 in, 1 out]
                  n259 = call-generic <vilib>:"NIMS_Get Any Vector_w Error - Matrix.vi"("A"=w621) -> ("Error Enum"=w606:T1, "Vector"=w623:dbl[])  [unwired: 8 in, 1 out]
                  n260 = call-generic <vilib>:"NIMS_Get Row Vector_w Error - Matrix.vi"("A"=w626) -> ("Error Enum"=w609:T1, "Row Vector"=w625:T2[])  [unwired: 8 in, 1 out]
                  n261 = call <vilib>:"NIMS_CH_Character RV to String.vi"("Character array"=w625) -> ("String"=w627:string)  [unwired: 10 in]
                  n262 = call <vilib>:"NIMS_String to Enum.vi"("Input String"=w627, "Enum choices"=string[] ["minorder"] ("Enum Options")) -> ("Error Enum"=w608:T1, "Enum Index"=w628:i32)  [unwired: 8 in]
                  n263 = call <vilib>:"NIMS_DF_fir_linf(m, f, mag, ripple, tm).vi"("type"=w614, "ripple"=w617, "mag"=w620, "f"=w623, "flag"=w628) -> ("error"=w599:i32, "b"=w590:dbl[])  [unwired: 5 in]
                  n264 = Build Array(w593, w593, w593, w593, w593, w593, w593, w593, w593, w593, "fir_linf") -> (w596:string[])
                  n265 = Build Array(w609, w608, w607, w606, w605, w604, w603, w602, w601, w600, w599) -> (w597:i32[])
                  n266 = call <vilib>:"NIMS_Create Error From Enums.vi"("Error Code"=bool[] [FALSE, FALSE, FALSE, FALSE, FALSE, FALSE, FALSE, FALSE, FALSE, FALSE, TRUE], "error in (no error)"=w595, "Line no"=w598, "Error Enums"=w597, "Function names"=w596) -> ("error out"=w591:errorcluster)  [unwired: 6 in]
                }
              }
              n267 = Build Array(w524) -> (w523:dbl[][])
              n268 = To Double Precision Complex(1:w523) -> (0:w522:cdb[][])
              n269 = call-generic <vilib>:"NIMS_RunTimeType_From StrictType (excl LVString).vi"("Plug-In Name"="", "Data In"=w522) -> ("Data Out"=w520:variant)  [unwired: 2 in]
              n270 = Build Array(w520) -> (w519:variant[])
            }
          }
        }
        frame 6 {
          n271 = case shown="1" w629 {
            tunnel: [_ w641 w763] -> w635
            tunnel: w632 -> [w639 _ _]
            tunnel: w633 -> [w640 w673 w795]
            tunnel: w631 -> [w637 w671 w793]
            tunnel: [w636 w647 w769] -> w630
            tunnel: w634 -> [_ w674 w796]
            frame Default {
              n272 = call <vilib>:"Create Error.vi"("Function name"=w639, "error in (no error)"=w637, "Error Enum"=error."Wrong number of output arguments", "Line number"=w640) -> ("error out"=w636:errorcluster)  [unwired: 6 in, 1 out]
            }
            frame 0 {
              n273 = Index Array(array=w674) -> (element #1=w670:variant, element #2=w665:variant, element #3=w661:variant, element #4=w657:variant, element #5=w653:variant, element #6=w650:variant)  [unwired: 6 in]
              n274 = call <vilib>:"NIMS_RunTimeType_Get Case Value.vi"("Data In"=w650) -> ("Case Value"=w648:string)  [unwired: 9 in, 1 out]
              n275 = call <vilib>:"NIMS_CH_RunTimeType_To Character 2D.vi"("Variant"=w650) -> ("data"=w649:T2[][])  [unwired: 1 in]
              n276 = call <vilib>:"NIMS_RunTimeType_Get Case Value.vi"("Data In"=w653) -> ("Case Value"=w651:string)  [unwired: 9 in, 1 out]
              n277 = call <vilib>:"NIMS_CH_RunTimeType_To Character 2D.vi"("Variant"=w653) -> ("data"=w652:T2[][])  [unwired: 1 in]
              n278 = call <vilib>:"NIMS_RunTimeType_Get Case Value.vi"("Data In"=w657) -> ("Case Value"=w654:string)  [unwired: 9 in, 1 out]
              n279 = call-generic <vilib>:"NIMS_RunTimeType_To Numeric.vi"("DataType"=cdb[][] [], "Variant"=w657) -> ("data"=w655:cdb[][])  [unwired: 1 in]
              n280 = call <vilib>:"NIMS_RunTimeType_Get Case Value.vi"("Data In"=w661) -> ("Case Value"=w658:string)  [unwired: 9 in, 1 out]
              n281 = call-generic <vilib>:"NIMS_RunTimeType_To Numeric.vi"("DataType"=cdb[][] [], "Variant"=w661) -> ("data"=w659:cdb[][])  [unwired: 1 in]
              n282 = call <vilib>:"NIMS_RunTimeType_Get Case Value.vi"("Data In"=w665) -> ("Case Value"=w662:string)  [unwired: 9 in, 1 out]
              n283 = call-generic <vilib>:"NIMS_RunTimeType_To Numeric.vi"("DataType"=cdb[][] [], "Variant"=w665) -> ("data"=w663:cdb[][])  [unwired: 1 in]
              n284 = call <vilib>:"NIMS_RunTimeType_Get Case Value.vi"("Data In"=w670) -> ("Case Value"=w666:string)  [unwired: 9 in, 1 out]
              n285 = call <vilib>:"NIMS_CH_RunTimeType_To Character 2D.vi"("Variant"=w670) -> ("data"=w667:T2[][])  [unwired: 1 in]
              n286 = call-generic <vilib>:"NIMS_RunTimeType_To Numeric.vi"("DataType"=cdb[][] [], "Variant"=w670) -> ("data"=w668:cdb[][])  [unwired: 1 in]
              n287 = Concatenate Strings(w666, w662, w658, w654, w651, w648) -> (w672:string)
              n288 = case shown="\"_Char:Character;;;;_Char:Character;_Char:Character;\"" w672 {
                tunnel: w671 -> [w676 w685 w727]
                tunnel: [_ w680 w722] -> w646
                tunnel: [w675 w681 w723] -> w647
                tunnel: w668 -> [_ w720 _]
                tunnel: w667 -> [_ _ w761]
                tunnel: w663 -> [_ w716 w757]
                tunnel: w659 -> [_ w713 w754]
                tunnel: w655 -> [_ w710 w751]
                tunnel: w652 -> [_ w707 w748]
                tunnel: w649 -> [_ w703 w744]
                tunnel: w673 -> [w679 w688 w730]
                frame Default {
                  n289 = call <vilib>:"Create Error.vi"("Function name"="fir_linf", "error in (no error)"=w676, "Error Enum"=23, "Line number"=w679) -> ("error out"=w675:errorcluster)  [unwired: 6 in, 1 out]
                }
                frame ";;;;_Char:Character;_Char:Character;" {
                  w683 = "fir_linf"
                  n290 = call-generic <vilib>:"NIMS_Get Row Vector_w Error - Matrix.vi"("A"=w703) -> ("Error Enum"=w691:T1, "Row Vector"=w702:T2[])  [unwired: 8 in, 1 out]
                  n291 = call <vilib>:"NIMS_CH_Character RV to String.vi"("Character array"=w702) -> ("String"=w704:string)  [unwired: 10 in]
                  n292 = call <vilib>:"NIMS_String to Enum.vi"("Input String"=w704, "Enum choices"=string[] ["hilbert", "differentiator", "minphase", "maxphase"] ("Enum Options")) -> ("Error Enum"=w690:T1, "Enum Index"=w705:i32)  [unwired: 8 in]
                  n293 = call-generic <vilib>:"NIMS_Get Row Vector_w Error - Matrix.vi"("A"=w707) -> ("Error Enum"=w692:T1, "Row Vector"=w706:T2[])  [unwired: 8 in, 1 out]
                  n294 = call <vilib>:"NIMS_CH_Character RV to String.vi"("Character array"=w706) -> ("String"=w708:string)  [unwired: 10 in]
                  n295 = call-generic <vilib>:"NIMS_Complex To Real.vi"("A"=w710) -> ("Error Enum"=w694:T1, "Real(A)"=w709:dbl[][])  [unwired: 8 in, 1 out]
                  n296 = call-generic <vilib>:"NIMS_Get Any Vector_w Error - Matrix.vi"("A"=w709) -> ("Error Enum"=w693:T1, "Vector"=w711:dbl[])  [unwired: 8 in, 1 out]
                  n297 = call-generic <vilib>:"NIMS_Complex To Real.vi"("A"=w713) -> ("Error Enum"=w696:T1, "Real(A)"=w712:dbl[][])  [unwired: 8 in, 1 out]
                  n298 = call-generic <vilib>:"NIMS_Get Any Vector_w Error - Matrix.vi"("A"=w712) -> ("Error Enum"=w695:T1, "Vector"=w714:dbl[])  [unwired: 8 in, 1 out]
                  n299 = call-generic <vilib>:"NIMS_Complex To Real.vi"("A"=w716) -> ("Error Enum"=w698:T1, "Real(A)"=w715:dbl[][])  [unwired: 8 in, 1 out]
                  n300 = call-generic <vilib>:"NIMS_Get Any Vector_w Error - Matrix.vi"("A"=w715) -> ("Error Enum"=w697:T1, "Vector"=w717:dbl[])  [unwired: 8 in, 1 out]
                  n301 = call-generic <vilib>:"NIMS_Complex To Real.vi"("A"=w720) -> ("Error Enum"=w700:T1, "Real(A)"=w719:dbl[][])  [unwired: 8 in, 1 out]
                  n302 = To Long Integer(number=w719) -> (32bit integer=w718:i32[][])
                  n303 = call-generic <vilib>:"NIMS_Get Scalar_w Error.vi"("A"=w718) -> ("Error Enum"=w699:T1, "Scalar"=w721:i32)  [unwired: 8 in, 1 out]
                  n304 = call <vilib>:"NIMS_DF_fir_linf(n, f, mag, w, ftype, t).vi"("t"=w705, "ftype"=w708, "w"=w711, "mag"=w714, "f"=w717, "n"=w721) -> ("error"=w689:i32, "b"=w680:dbl[])  [unwired: 4 in]
                  n305 = Build Array(w683, w683, w683, w683, w683, w683, w683, w683, w683, w683, w683, "fir_linf") -> (w686:string[])
                  n306 = Build Array(w700, w699, w698, w697, w696, w695, w694, w693, w692, w691, w690, w689) -> (w687:i32[])
                  n307 = call <vilib>:"NIMS_Create Error From Enums.vi"("Error Code"=bool[] [FALSE, FALSE, FALSE, FALSE, FALSE, FALSE, FALSE, FALSE, FALSE, FALSE, FALSE, TRUE], "error in (no error)"=w685, "Line no"=w688, "Error Enums"=w687, "Function names"=w686) -> ("error out"=w681:errorcluster)  [unwired: 6 in]
                }
                frame "_Char:Character;;;;_Char:Character;_Char:Character;" {
                  w725 = "fir_linf"
                  n308 = call-generic <vilib>:"NIMS_Get Row Vector_w Error - Matrix.vi"("A"=w744) -> ("Error Enum"=w733:T1, "Row Vector"=w743:T2[])  [unwired: 8 in, 1 out]
                  n309 = call <vilib>:"NIMS_CH_Character RV to String.vi"("Character array"=w743) -> ("String"=w745:string)  [unwired: 10 in]
                  n310 = call <vilib>:"NIMS_String to Enum.vi"("Input String"=w745, "Enum choices"=string[] ["hilbert", "differentiator", "minphase", "maxphase"] ("Enum Options")) -> ("Error Enum"=w732:T1, "Enum Index"=w746:i32)  [unwired: 8 in]
                  n311 = call-generic <vilib>:"NIMS_Get Row Vector_w Error - Matrix.vi"("A"=w748) -> ("Error Enum"=w734:T1, "Row Vector"=w747:T2[])  [unwired: 8 in, 1 out]
                  n312 = call <vilib>:"NIMS_CH_Character RV to String.vi"("Character array"=w747) -> ("String"=w749:string)  [unwired: 10 in]
                  n313 = call-generic <vilib>:"NIMS_Complex To Real.vi"("A"=w751) -> ("Error Enum"=w736:T1, "Real(A)"=w750:dbl[][])  [unwired: 8 in, 1 out]
                  n314 = call-generic <vilib>:"NIMS_Get Any Vector_w Error - Matrix.vi"("A"=w750) -> ("Error Enum"=w735:T1, "Vector"=w752:dbl[])  [unwired: 8 in, 1 out]
                  n315 = call-generic <vilib>:"NIMS_Complex To Real.vi"("A"=w754) -> ("Error Enum"=w738:T1, "Real(A)"=w753:dbl[][])  [unwired: 8 in, 1 out]
                  n316 = call-generic <vilib>:"NIMS_Get Any Vector_w Error - Matrix.vi"("A"=w753) -> ("Error Enum"=w737:T1, "Vector"=w755:dbl[])  [unwired: 8 in, 1 out]
                  n317 = call-generic <vilib>:"NIMS_Complex To Real.vi"("A"=w757) -> ("Error Enum"=w740:T1, "Real(A)"=w756:dbl[][])  [unwired: 8 in, 1 out]
                  n318 = call-generic <vilib>:"NIMS_Get Any Vector_w Error - Matrix.vi"("A"=w756) -> ("Error Enum"=w739:T1, "Vector"=w758:dbl[])  [unwired: 8 in, 1 out]
                  n319 = call <vilib>:"NIMS_CH_Character 2D to U8 2D.vi"("Character 2D array"=w761) -> ("U8 2D array"=w760:u8[][])  [unwired: 10 in]
                  n320 = To Long Integer(number=w760) -> (32bit integer=w759:i32[][])
                  n321 = call-generic <vilib>:"NIMS_Get Scalar_w Error.vi"("A"=w759) -> ("Error Enum"=w741:T1, "Scalar"=w762:i32)  [unwired: 8 in, 1 out]
                  n322 = call <vilib>:"NIMS_DF_fir_linf(n, f, mag, w, ftype, t).vi"("t"=w746, "ftype"=w749, "w"=w752, "mag"=w755, "f"=w758, "n"=w762) -> ("error"=w731:i32, "b"=w722:dbl[])  [unwired: 4 in]
                  n323 = Build Array(w725, w725, w725, w725, w725, w725, w725, w725, w725, w725, "fir_linf") -> (w728:string[])
                  n324 = Build Array(w741, w740, w739, w738, w737, w736, w735, w734, w733, w732, w731) -> (w729:i32[])
                  n325 = call <vilib>:"NIMS_Create Error From Enums.vi"("Error Code"=bool[] [FALSE, FALSE, FALSE, FALSE, FALSE, FALSE, FALSE, FALSE, FALSE, FALSE, TRUE], "error in (no error)"=w727, "Line no"=w730, "Error Enums"=w729, "Function names"=w728) -> ("error out"=w723:errorcluster)  [unwired: 6 in]
                }
              }
              n326 = Build Array(w646) -> (w645:dbl[][])
              n327 = To Double Precision Complex(1:w645) -> (0:w644:cdb[][])
              n328 = call-generic <vilib>:"NIMS_RunTimeType_From StrictType (excl LVString).vi"("Plug-In Name"="", "Data In"=w644) -> ("Data Out"=w642:variant)  [unwired: 2 in]
              n329 = Build Array(w642) -> (w641:variant[])
            }
            frame 1 {
              n330 = Index Array(array=w796) -> (element #1=w792:variant, element #2=w787:variant, element #3=w783:variant, element #4=w779:variant, element #5=w775:variant, element #6=w772:variant)  [unwired: 6 in]
              n331 = call <vilib>:"NIMS_RunTimeType_Get Case Value.vi"("Data In"=w772) -> ("Case Value"=w770:string)  [unwired: 9 in, 1 out]
              n332 = call <vilib>:"NIMS_CH_RunTimeType_To Character 2D.vi"("Variant"=w772) -> ("data"=w771:T2[][])  [unwired: 1 in]
              n333 = call <vilib>:"NIMS_RunTimeType_Get Case Value.vi"("Data In"=w775) -> ("Case Value"=w773:string)  [unwired: 9 in, 1 out]
              n334 = call <vilib>:"NIMS_CH_RunTimeType_To Character 2D.vi"("Variant"=w775) -> ("data"=w774:T2[][])  [unwired: 1 in]
              n335 = call <vilib>:"NIMS_RunTimeType_Get Case Value.vi"("Data In"=w779) -> ("Case Value"=w776:string)  [unwired: 9 in, 1 out]
              n336 = call-generic <vilib>:"NIMS_RunTimeType_To Numeric.vi"("DataType"=cdb[][] [], "Variant"=w779) -> ("data"=w777:cdb[][])  [unwired: 1 in]
              n337 = call <vilib>:"NIMS_RunTimeType_Get Case Value.vi"("Data In"=w783) -> ("Case Value"=w780:string)  [unwired: 9 in, 1 out]
              n338 = call-generic <vilib>:"NIMS_RunTimeType_To Numeric.vi"("DataType"=cdb[][] [], "Variant"=w783) -> ("data"=w781:cdb[][])  [unwired: 1 in]
              n339 = call <vilib>:"NIMS_RunTimeType_Get Case Value.vi"("Data In"=w787) -> ("Case Value"=w784:string)  [unwired: 9 in, 1 out]
              n340 = call-generic <vilib>:"NIMS_RunTimeType_To Numeric.vi"("DataType"=cdb[][] [], "Variant"=w787) -> ("data"=w785:cdb[][])  [unwired: 1 in]
              n341 = call <vilib>:"NIMS_RunTimeType_Get Case Value.vi"("Data In"=w792) -> ("Case Value"=w788:string)  [unwired: 9 in, 1 out]
              n342 = call <vilib>:"NIMS_CH_RunTimeType_To Character 2D.vi"("Variant"=w792) -> ("data"=w789:T2[][])  [unwired: 1 in]
              n343 = call-generic <vilib>:"NIMS_RunTimeType_To Numeric.vi"("DataType"=cdb[][] [], "Variant"=w792) -> ("data"=w790:cdb[][])  [unwired: 1 in]
              n344 = Concatenate Strings(w788, w784, w780, w776, w773, w770) -> (w794:string)
              n345 = case shown="\"_Char:Character;;;;_Char:Character;_Char:Character;\"" w794 {
                tunnel: w793 -> [w798 w807 w849]
                tunnel: [_ w802 w844] -> w768
                tunnel: [w797 w803 w845] -> w769
                tunnel: w790 -> [_ w842 _]
                tunnel: w789 -> [_ _ w883]
                tunnel: w785 -> [_ w838 w879]
                tunnel: w781 -> [_ w835 w876]
                tunnel: w777 -> [_ w832 w873]
                tunnel: w774 -> [_ w829 w870]
                tunnel: w771 -> [_ w825 w866]
                tunnel: w795 -> [w801 w810 w852]
                frame Default {
                  n346 = call <vilib>:"Create Error.vi"("Function name"="fir_linf", "error in (no error)"=w798, "Error Enum"=23, "Line number"=w801) -> ("error out"=w797:errorcluster)  [unwired: 6 in, 1 out]
                }
                frame ";;;;_Char:Character;_Char:Character;" {
                  w805 = "fir_linf"
                  n347 = call-generic <vilib>:"NIMS_Get Row Vector_w Error - Matrix.vi"("A"=w825) -> ("Error Enum"=w813:T1, "Row Vector"=w824:T2[])  [unwired: 8 in, 1 out]
                  n348 = call <vilib>:"NIMS_CH_Character RV to String.vi"("Character array"=w824) -> ("String"=w826:string)  [unwired: 10 in]
                  n349 = call <vilib>:"NIMS_String to Enum.vi"("Input String"=w826, "Enum choices"=string[] ["hilbert", "differentiator", "minphase", "maxphase"] ("Enum Options")) -> ("Error Enum"=w812:T1, "Enum Index"=w827:i32)  [unwired: 8 in]
                  n350 = call-generic <vilib>:"NIMS_Get Row Vector_w Error - Matrix.vi"("A"=w829) -> ("Error Enum"=w814:T1, "Row Vector"=w828:T2[])  [unwired: 8 in, 1 out]
                  n351 = call <vilib>:"NIMS_CH_Character RV to String.vi"("Character array"=w828) -> ("String"=w830:string)  [unwired: 10 in]
                  n352 = call-generic <vilib>:"NIMS_Complex To Real.vi"("A"=w832) -> ("Error Enum"=w816:T1, "Real(A)"=w831:dbl[][])  [unwired: 8 in, 1 out]
                  n353 = call-generic <vilib>:"NIMS_Get Any Vector_w Error - Matrix.vi"("A"=w831) -> ("Error Enum"=w815:T1, "Vector"=w833:dbl[])  [unwired: 8 in, 1 out]
                  n354 = call-generic <vilib>:"NIMS_Complex To Real.vi"("A"=w835) -> ("Error Enum"=w818:T1, "Real(A)"=w834:dbl[][])  [unwired: 8 in, 1 out]
                  n355 = call-generic <vilib>:"NIMS_Get Any Vector_w Error - Matrix.vi"("A"=w834) -> ("Error Enum"=w817:T1, "Vector"=w836:dbl[])  [unwired: 8 in, 1 out]
                  n356 = call-generic <vilib>:"NIMS_Complex To Real.vi"("A"=w838) -> ("Error Enum"=w820:T1, "Real(A)"=w837:dbl[][])  [unwired: 8 in, 1 out]
                  n357 = call-generic <vilib>:"NIMS_Get Any Vector_w Error - Matrix.vi"("A"=w837) -> ("Error Enum"=w819:T1, "Vector"=w839:dbl[])  [unwired: 8 in, 1 out]
                  n358 = call-generic <vilib>:"NIMS_Complex To Real.vi"("A"=w842) -> ("Error Enum"=w822:T1, "Real(A)"=w841:dbl[][])  [unwired: 8 in, 1 out]
                  n359 = To Long Integer(number=w841) -> (32bit integer=w840:i32[][])
                  n360 = call-generic <vilib>:"NIMS_Get Scalar_w Error.vi"("A"=w840) -> ("Error Enum"=w821:T1, "Scalar"=w843:i32)  [unwired: 8 in, 1 out]
                  n361 = call <vilib>:"NIMS_DF_fir_linf(n, f, mag, w, ftype, t).vi"("t"=w827, "ftype"=w830, "w"=w833, "mag"=w836, "f"=w839, "n"=w843) -> ("error"=w811:i32, "b"=w802:dbl[])  [unwired: 4 in]
                  n362 = Build Array(w805, w805, w805, w805, w805, w805, w805, w805, w805, w805, w805, "fir_linf") -> (w808:string[])
                  n363 = Build Array(w822, w821, w820, w819, w818, w817, w816, w815, w814, w813, w812, w811) -> (w809:i32[])
                  n364 = call <vilib>:"NIMS_Create Error From Enums.vi"("Error Code"=bool[] [FALSE, FALSE, FALSE, FALSE, FALSE, FALSE, FALSE, FALSE, FALSE, FALSE, FALSE, TRUE], "error in (no error)"=w807, "Line no"=w810, "Error Enums"=w809, "Function names"=w808) -> ("error out"=w803:errorcluster)  [unwired: 6 in]
                }
                frame "_Char:Character;;;;_Char:Character;_Char:Character;" {
                  w847 = "fir_linf"
                  n365 = call-generic <vilib>:"NIMS_Get Row Vector_w Error - Matrix.vi"("A"=w866) -> ("Error Enum"=w855:T1, "Row Vector"=w865:T2[])  [unwired: 8 in, 1 out]
                  n366 = call <vilib>:"NIMS_CH_Character RV to String.vi"("Character array"=w865) -> ("String"=w867:string)  [unwired: 10 in]
                  n367 = call <vilib>:"NIMS_String to Enum.vi"("Input String"=w867, "Enum choices"=string[] ["hilbert", "differentiator", "minphase", "maxphase"] ("Enum Options")) -> ("Error Enum"=w854:T1, "Enum Index"=w868:i32)  [unwired: 8 in]
                  n368 = call-generic <vilib>:"NIMS_Get Row Vector_w Error - Matrix.vi"("A"=w870) -> ("Error Enum"=w856:T1, "Row Vector"=w869:T2[])  [unwired: 8 in, 1 out]
                  n369 = call <vilib>:"NIMS_CH_Character RV to String.vi"("Character array"=w869) -> ("String"=w871:string)  [unwired: 10 in]
                  n370 = call-generic <vilib>:"NIMS_Complex To Real.vi"("A"=w873) -> ("Error Enum"=w858:T1, "Real(A)"=w872:dbl[][])  [unwired: 8 in, 1 out]
                  n371 = call-generic <vilib>:"NIMS_Get Any Vector_w Error - Matrix.vi"("A"=w872) -> ("Error Enum"=w857:T1, "Vector"=w874:dbl[])  [unwired: 8 in, 1 out]
                  n372 = call-generic <vilib>:"NIMS_Complex To Real.vi"("A"=w876) -> ("Error Enum"=w860:T1, "Real(A)"=w875:dbl[][])  [unwired: 8 in, 1 out]
                  n373 = call-generic <vilib>:"NIMS_Get Any Vector_w Error - Matrix.vi"("A"=w875) -> ("Error Enum"=w859:T1, "Vector"=w877:dbl[])  [unwired: 8 in, 1 out]
                  n374 = call-generic <vilib>:"NIMS_Complex To Real.vi"("A"=w879) -> ("Error Enum"=w862:T1, "Real(A)"=w878:dbl[][])  [unwired: 8 in, 1 out]
                  n375 = call-generic <vilib>:"NIMS_Get Any Vector_w Error - Matrix.vi"("A"=w878) -> ("Error Enum"=w861:T1, "Vector"=w880:dbl[])  [unwired: 8 in, 1 out]
                  n376 = call <vilib>:"NIMS_CH_Character 2D to U8 2D.vi"("Character 2D array"=w883) -> ("U8 2D array"=w882:u8[][])  [unwired: 10 in]
                  n377 = To Long Integer(number=w882) -> (32bit integer=w881:i32[][])
                  n378 = call-generic <vilib>:"NIMS_Get Scalar_w Error.vi"("A"=w881) -> ("Error Enum"=w863:T1, "Scalar"=w884:i32)  [unwired: 8 in, 1 out]
                  n379 = call <vilib>:"NIMS_DF_fir_linf(n, f, mag, w, ftype, t).vi"("t"=w868, "ftype"=w871, "w"=w874, "mag"=w877, "f"=w880, "n"=w884) -> ("error"=w853:i32, "b"=w844:dbl[])  [unwired: 4 in]
                  n380 = Build Array(w847, w847, w847, w847, w847, w847, w847, w847, w847, w847, "fir_linf") -> (w850:string[])
                  n381 = Build Array(w863, w862, w861, w860, w859, w858, w857, w856, w855, w854, w853) -> (w851:i32[])
                  n382 = call <vilib>:"NIMS_Create Error From Enums.vi"("Error Code"=bool[] [FALSE, FALSE, FALSE, FALSE, FALSE, FALSE, FALSE, FALSE, FALSE, FALSE, TRUE], "error in (no error)"=w849, "Line no"=w852, "Error Enums"=w851, "Function names"=w850) -> ("error out"=w845:errorcluster)  [unwired: 6 in]
                }
              }
              n383 = Build Array(w768) -> (w767:dbl[][])
              n384 = To Double Precision Complex(1:w767) -> (0:w766:cdb[][])
              n385 = call-generic <vilib>:"NIMS_RunTimeType_From StrictType (excl LVString).vi"("Plug-In Name"="", "Data In"=w766) -> ("Data Out"=w764:variant)  [unwired: 2 in]
              n386 = Build Array(w764) -> (w763:variant[])
            }
          }
        }
      }
    }
    frame Error {
    }
  }
  "error out" <- w3
  "[funct(A)]" <- w4
